vi "GEA_ICP_SM.vi"(0 "ComPort":refnum<visa-resource-name>="COM1", 1 "Destination Address":u8=96 format="%.0x", 2 "Source Address":u8=128 format="%.0x", 5 "Command":u8(ring)=15 items=["CMD_WRITE_SETPOINTS", "RQST_NON_CRIT_VERSION", "RQST_CRIT_VERSION", "RQST_EEPROM_VERSION", "RQST_T2_RESISTANCE", "RQST_T3A_RESISTANCE", "RQST_T3B_RESISTANCE", "RQST_T4_RESISTANCE", "RQST_T5_RESISTANCE", "RQST_IDLB_RESISTANCE", "RQST_MODE_SELECT_RESISTANCE", "RQST_STATUS INFO", "RQST_SS_FAULT_COUNTS", "RQST_OTHER_FAULT_COUNTS", "CMD_CLEAR_FAULT_COUNTS", "RQST_HYPERTERM_OUTPUT_DATA", "RQST_READ_PERSONALITY", "RQST_DSM_OVERRIDE_STATUS", "RQST_STATUS_QUERY", "RQST_HEM_KWH_DATA", "RQST_SERVICE_ERROR_CODES", "RQST_OVERRIDE_STATUS", "CMD_CLEAR_OVERRIDE_STATUS", "CMD_CLEAR_ENERGY_USAGE_CTRS", "CMD_COMP_OFF", "CMD_UE_2_SECONDS", "CMD_LE_2_SECONDS", "CMD_COMP_ON", "CMD_HP_RUN_6MIN", "RQST_TEMP_RANGE", "RQST_VACATION_RANGE", "RQST_STD_ELEC_RANGE", "RQST_WATER_CAPACITY", "CMD_CANCEL_EEV_POSITION", "RQST_SUPPORTED_MODES", "CMD_CONTROL_FAN1", "CMD_EEV_POSITION", "CMD_SET_EEV_START_POSITION", "CMD_SET_EEV_STOP_POSITION", "CMD_UPDATE_DSM_LEVEL", "CMD_SET_PID_I_DENOMINATOR", "CMD_SET_PID_I_NUMERATOR", "RQST_DATA_FROM_MEMORY", "CMD_OVERRIDE_STATUS_CHANGED", "CMD_SET_PID_P_DENOMINATOR", "CMD_SET_PID_P_NUMERATOR", "CMD_SET_PID_RUN_SH_TARGET", "CMD_SET_PID_START_DWELL_TIME", "CMD_SET_PID_TRANSITION_TIME", "CMD_SET_PID_TRANS_SH_TARGET", "CMD_SET_PID_UPDATE_RATE", "RQST_DATA_FROM_DATA_FLASH", "CMD_DSM_OVERRIDES", "CMD_UPDATE_MODE", "CMD_UPDATE_SPECIAL_OPERATION", "CMD_SET_CURRENTS", "CMD_RESET_FILTER_TIMES", "CMD_TURN_ON_DLB", "RQST_PID_PARAMETERS", "CMD_CHECK_CRC", "CMD_ENTER_FACT_MODE", "CMD_RESET", "CMD_RESTORE_EEPROM_DEFAULTS"], 7 "Command Data":u8[](array[numeric]) format="%02x", 9 "InitSerial?":bool=TRUE, 11 "Error In":errorcluster) -> (4 "WriteACK":bool, 6 "Read_ACK":bool, 8 "DataReturned":u8[](array[numeric]) format="%.0x", 14 "CRC Match":bool, 15 "Error Out":errorcluster)   [LabVIEW 2009]
uses:
  <vilib>/Instr/_visa.llb/VISA Configure Serial Port (Instr).vi
  HEWH Error Enumeration.ctl
panel:
  in  "milliseconds to wait":u32=20
  out "Numeric":i32
  out "Serial Settings:Number of Bytes at Serial Port 4":u32
  out "byte count":u32=40
  out "Serial Settings:Number of Bytes at Serial Port 3":u32
  out "Serial Settings:Number of Bytes at Serial Port 2":u32
  out "tStart":u32
  out "Tdiff":i32[](array[numeric])
  out "Serial Settings:Number of Bytes at Serial Port":u32
  out "Time Array":i32[](array[numeric])
  out "ACK(E1?)":u8[](array[numeric]) format="%.0x"
  out "Local?":bool
  out "State Array":string[](array[string])
  out "CRCRead":u8[](array[numeric]) format="%.0x"
  out "Command":u8[](array[numeric])=[226, 96, 8, 128, 86, 123, 137, 227] format="%.0x"
  in  "Send HEWH Cmd":bool
  in  "Write Rand":bool
  in  "Random Data":u8[](array[numeric]) format="%.0x"
  out "WriteOK":bool
  out "ReadArray":u8[](array[numeric]) format="%.0x"
  in  "OK":bool
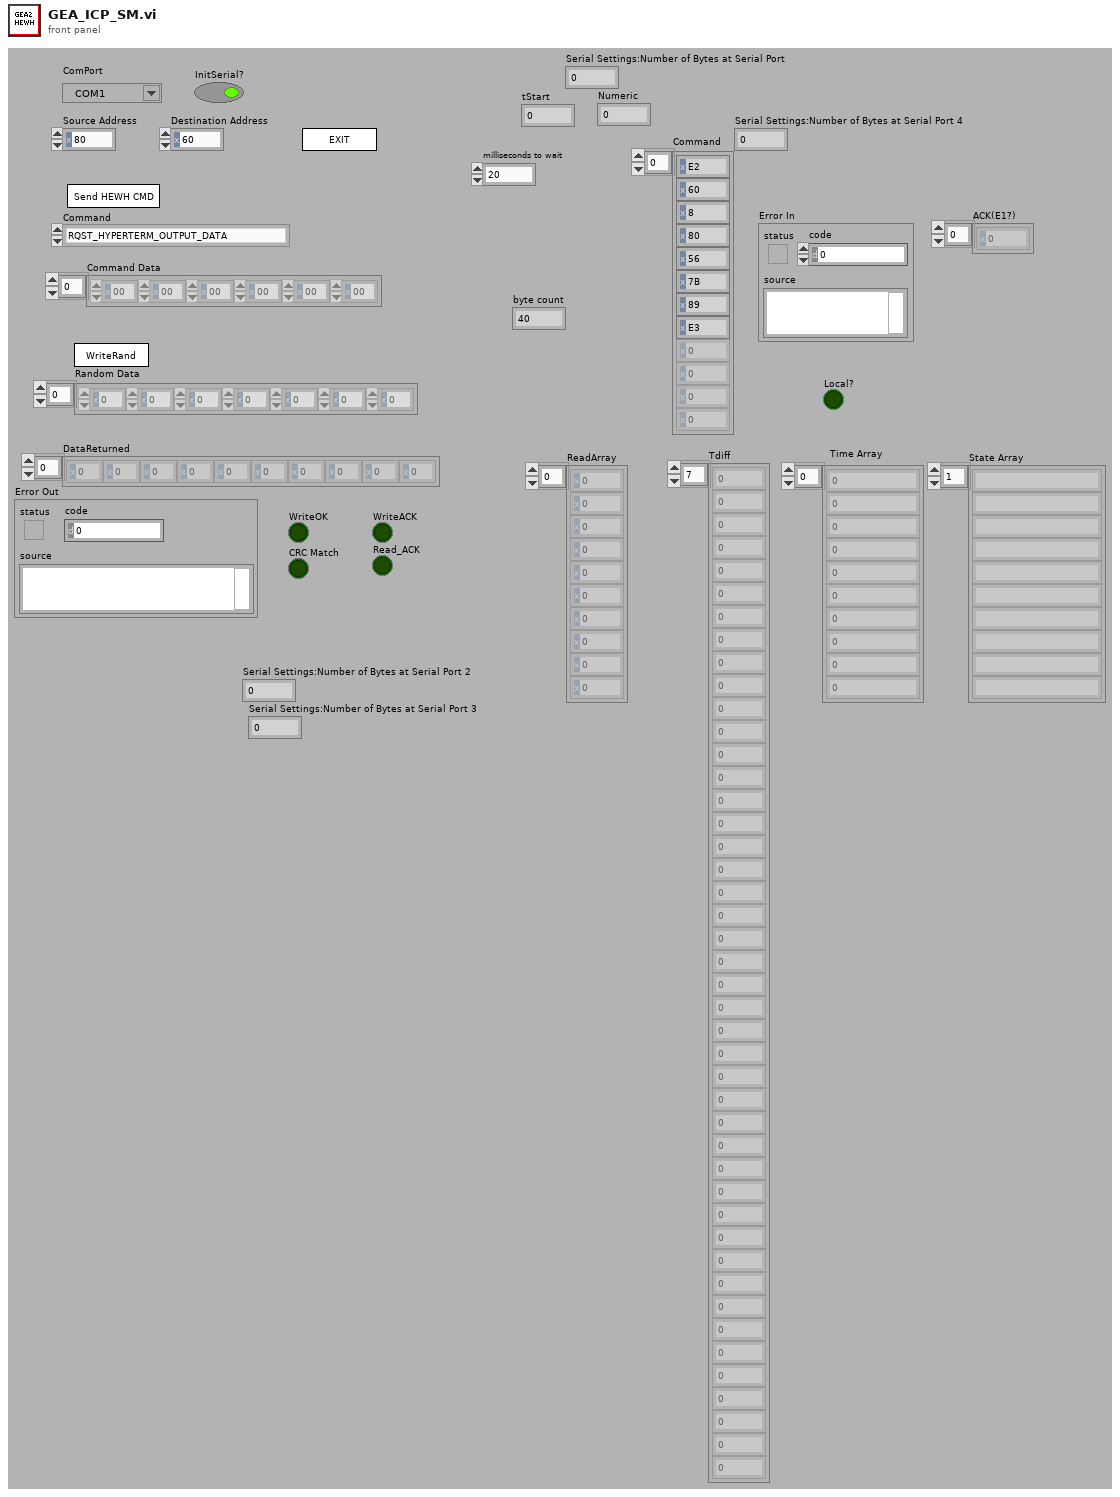
[diagram p1: front panel]
types:
  T1 = enum32{"invalid app kind", "Development System", "Run Time System", "Student Edition", "Embedded LabVIEW", "Evaluation", "Custom"}
  T2 = cluster{"Current VI Reference":refnum<vi>, "Close Panel on Exit?":bool}
  T3 = enum32{"Invalid", "Standard", "Closed", "Hidden", "Minimized", "Maximized"}
  T4 = typedef "HEWH Error Enumeration.ctl" = enum16{"No Error", "GEA2 Send ACK Mismatch", "GEA2 STX", "GEA2 ETX", "GEA2 CRC Mismatch", "GEA2 ReadACK", "RTD In Range Error", "Fail Mean Tank Temp", "No Flow Config Data Found", "Failed Flow During Purge", "Temp During Purge", "Confirm IF Stop Fail", "Init Draw: TC_1 Out of Range", "Flow = 0 During Draw after 20s"}
  T5 = cluster{"Core":cluster{"Current VI Reference":refnum<vi>, "Close Panel on Exit?":bool}, "ComPort":refnum<visa-resource-name>, "ReadArray":u8[], "CRCArray":u8[], "Bytes Remaining":u8, "CRCRead":u8[], "CRC":bool, "HEWH Command":u8, "Error Out Flag":bool, "Read Pos.":i32}
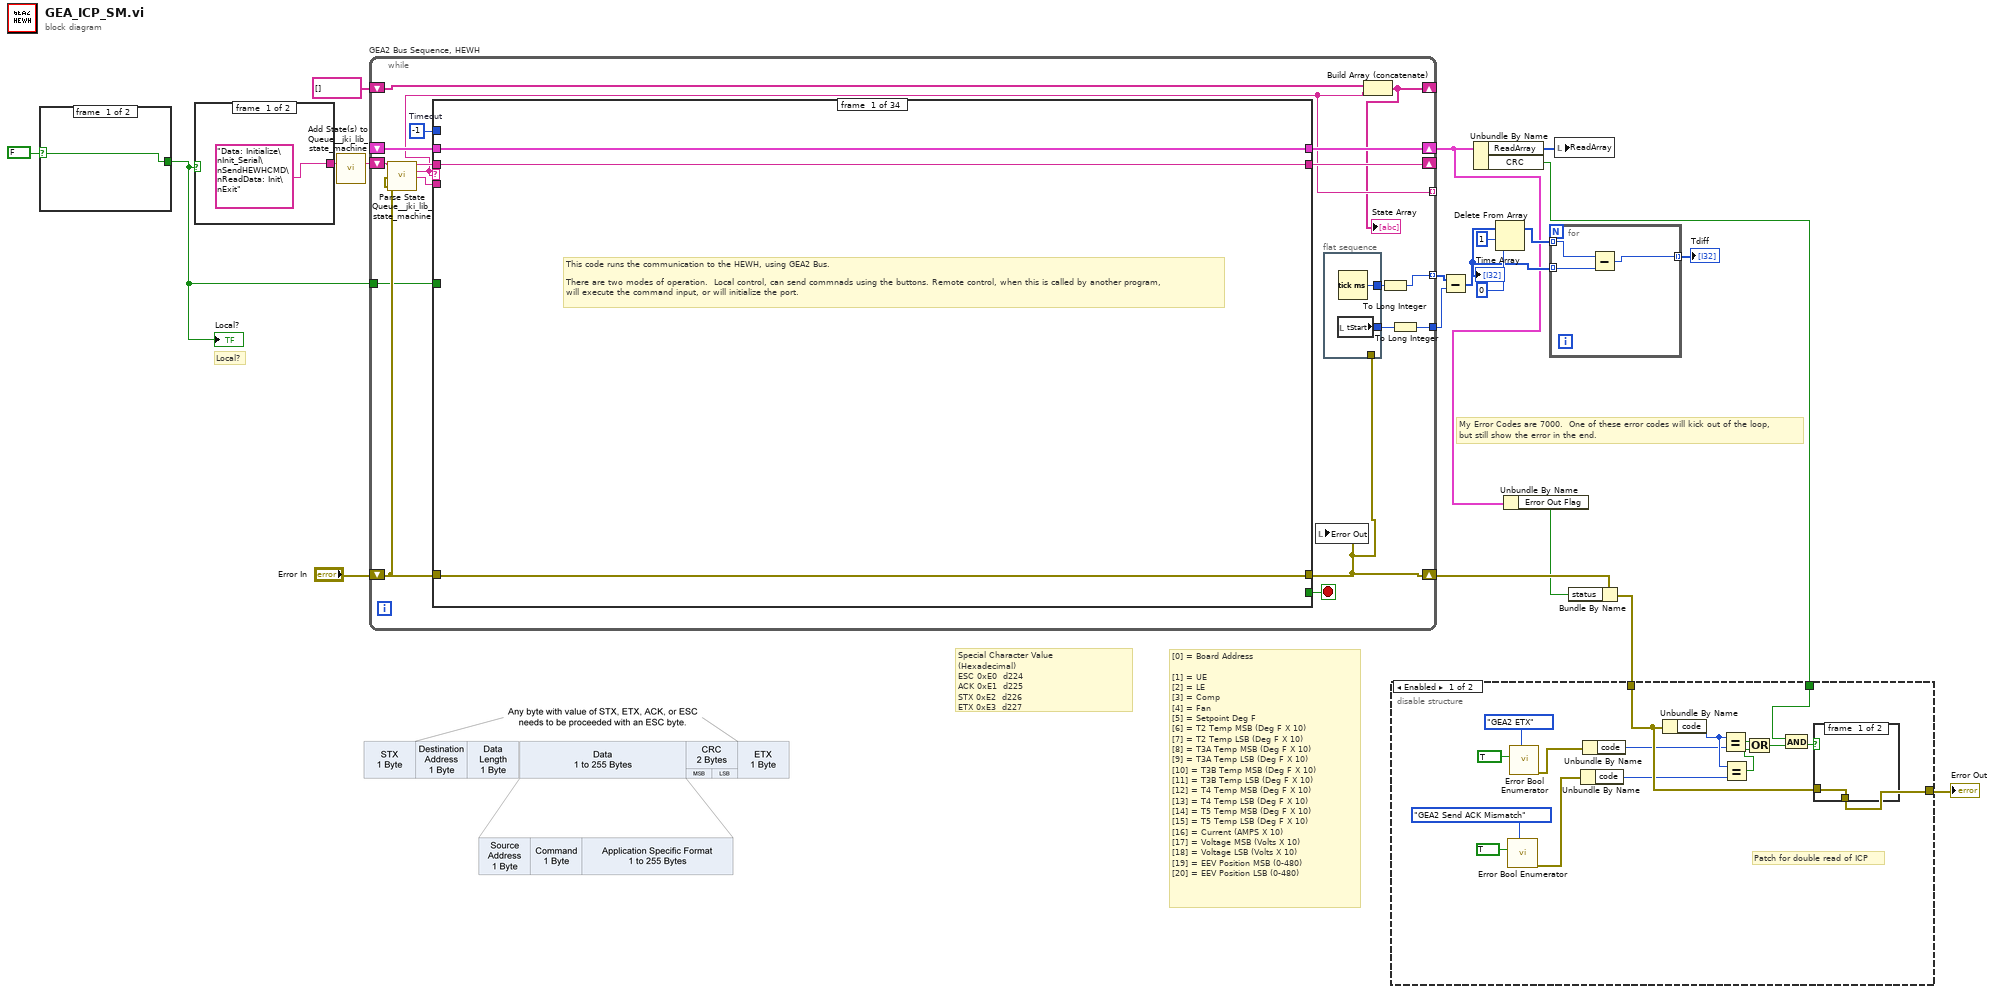
[diagram p0: block diagram]
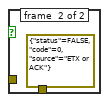
[diagram p2: hidden frame]
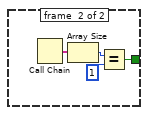
[diagram p4: hidden frame]
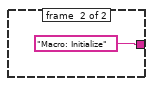
[diagram p5: hidden frame]
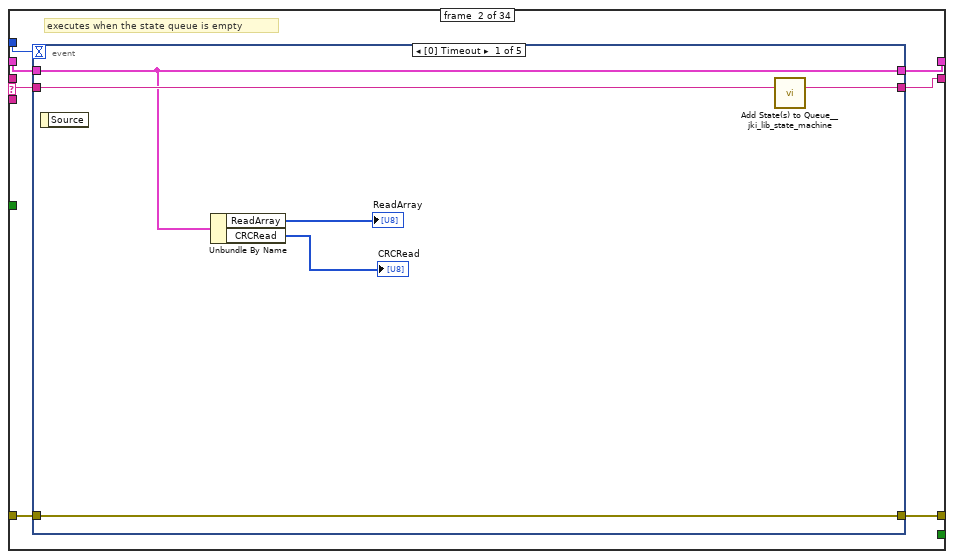
[diagram p6: hidden frame]
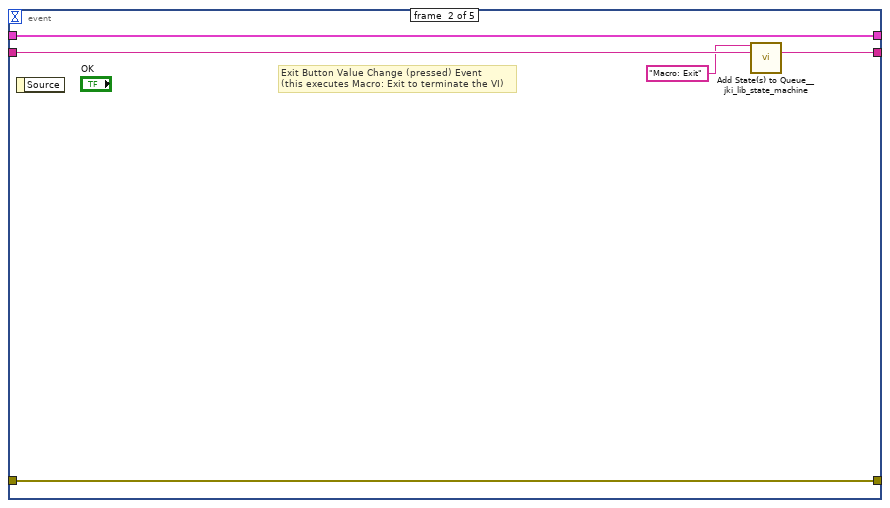
[diagram p7: hidden frame]
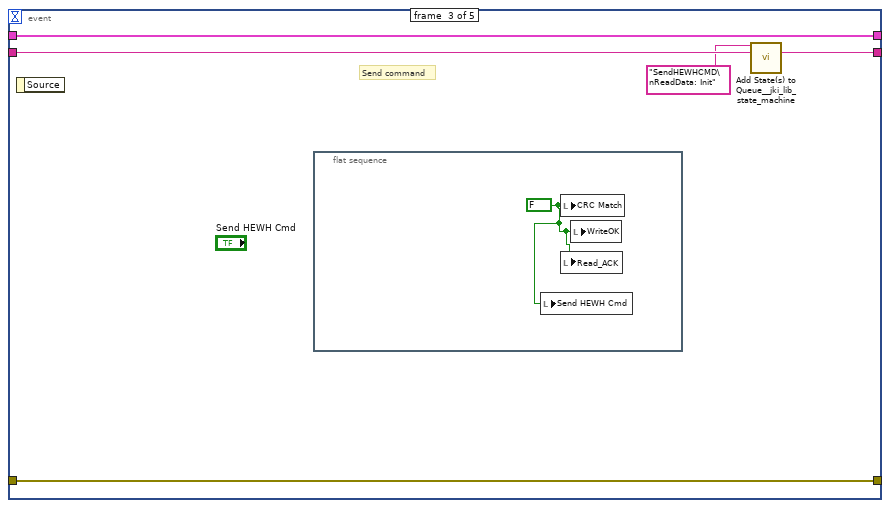
[diagram p8: hidden frame]
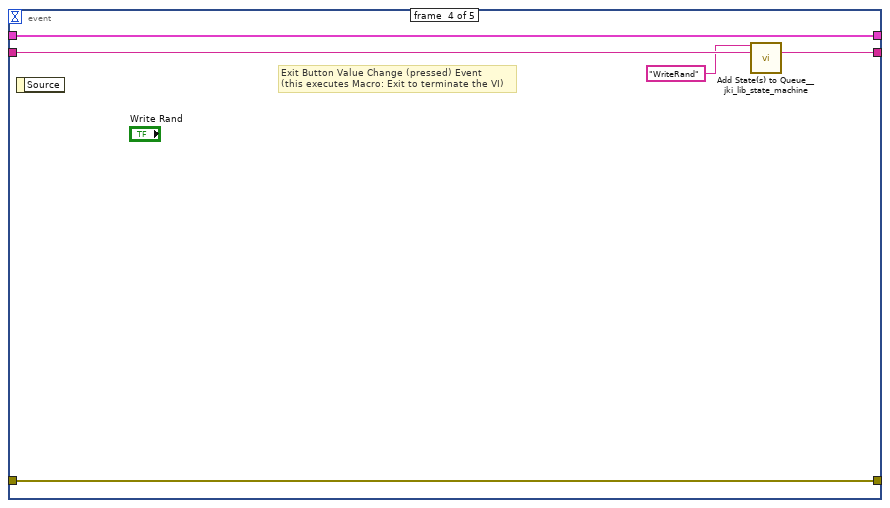
[diagram p9: hidden frame]
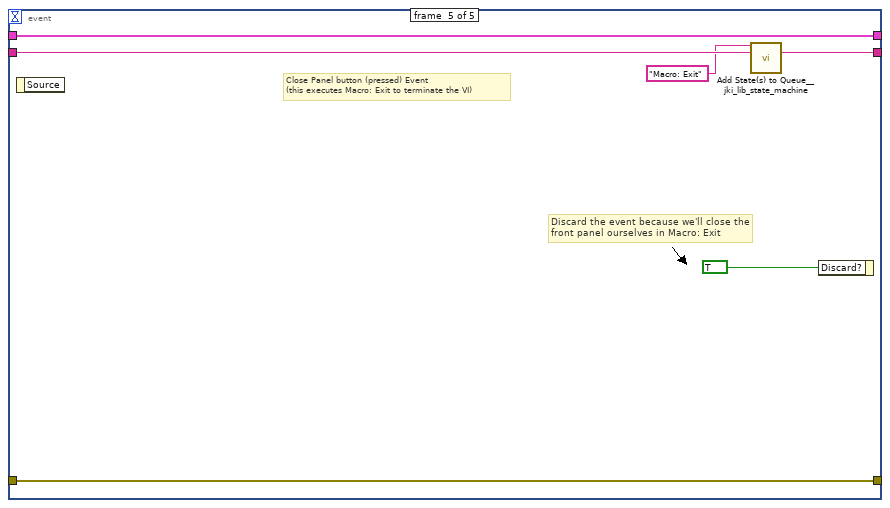
[diagram p10: hidden frame]
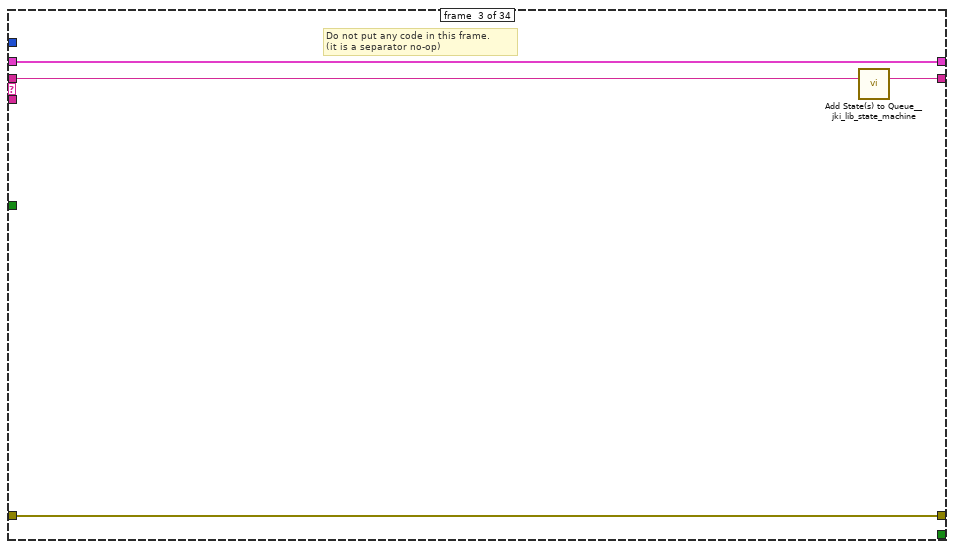
[diagram p11: hidden frame]
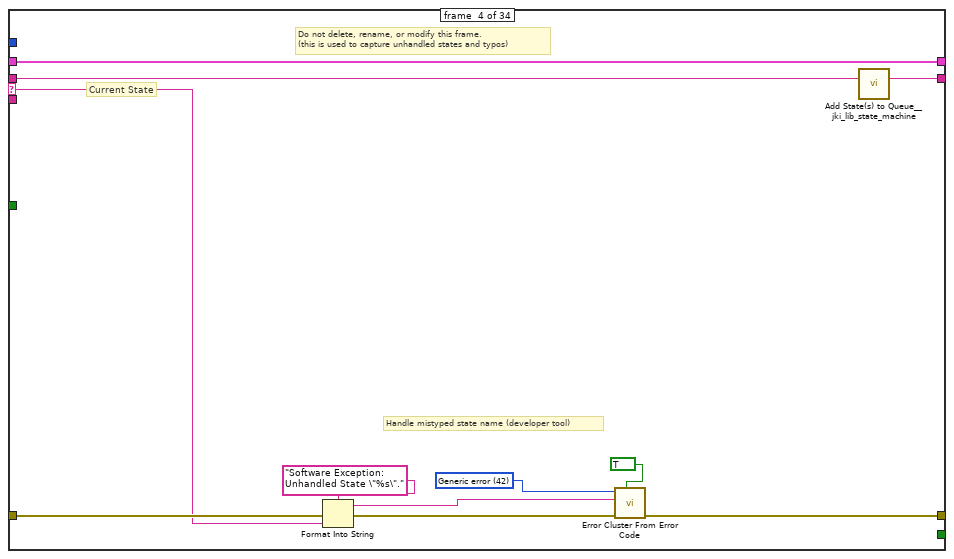
[diagram p12: hidden frame]
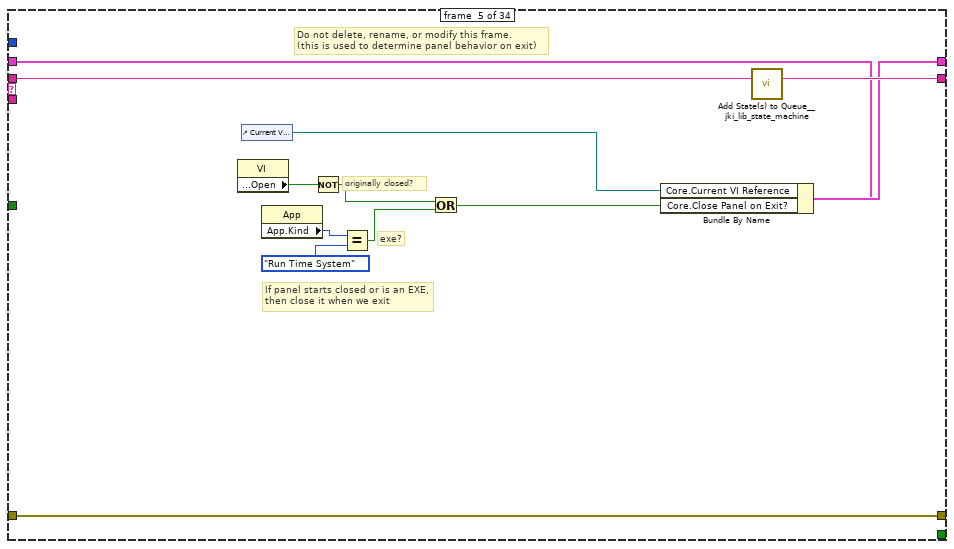
[diagram p13: hidden frame]
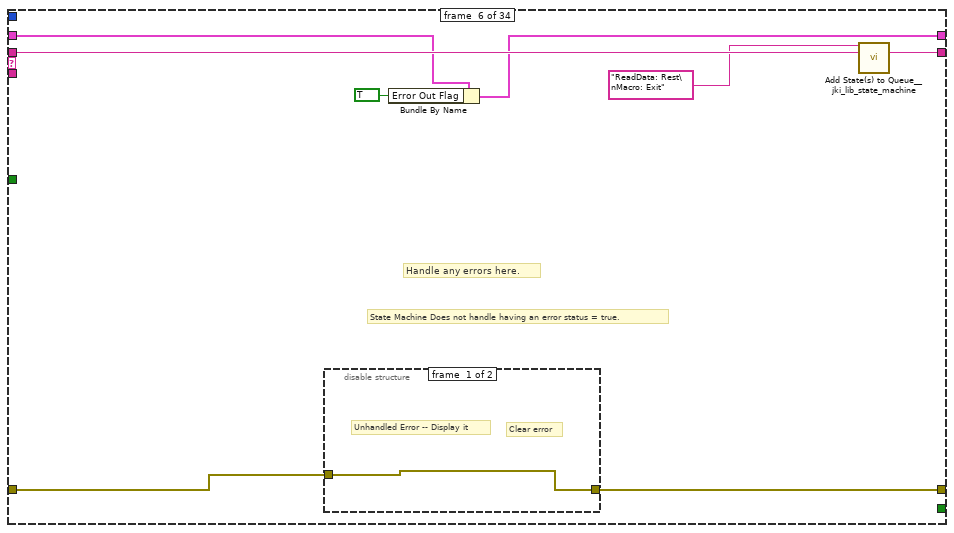
[diagram p14: hidden frame]
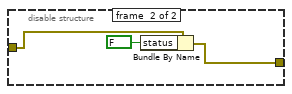
[diagram p15: hidden frame]
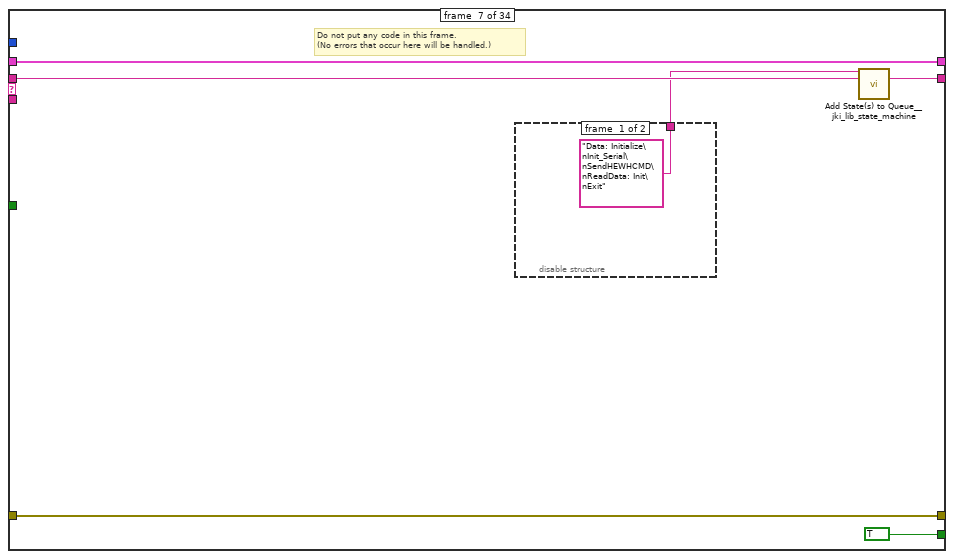
[diagram p16: hidden frame]
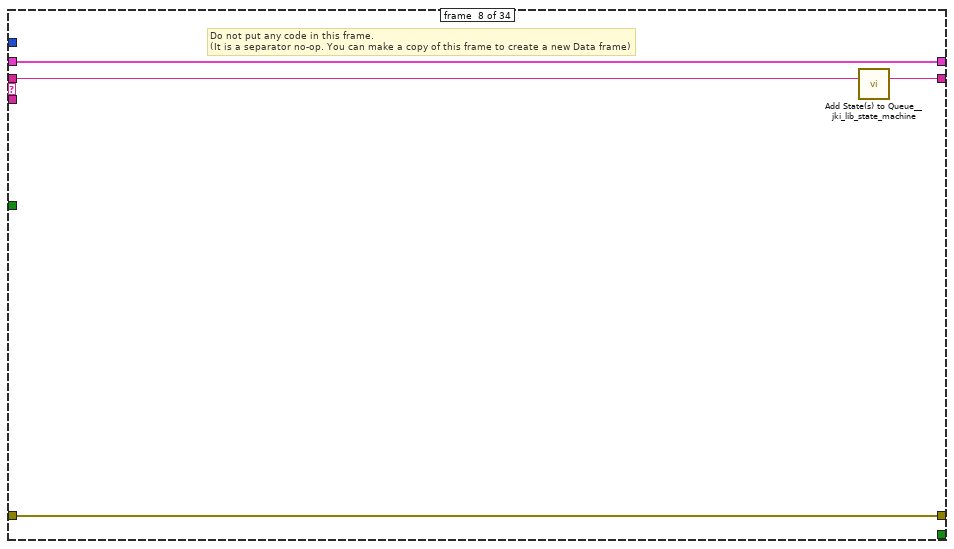
[diagram p18: hidden frame]
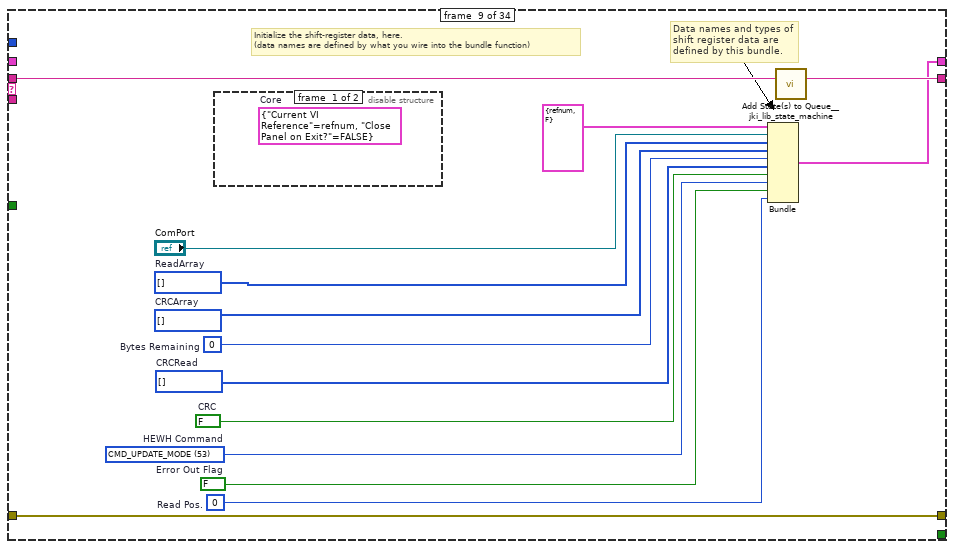
[diagram p19: hidden frame]
diagram:
  # "My Error Codes are 7000.  One of these error codes will kick out of the loop,\nbut still show the error in the end."
  # "Local?"
  # "Special Character\tValue (Hexadecimal)\nESC\t0xE0  d224\nACK\t0xE1  d225\nSTX\t0xE2  d226\nETX\t0xE3  d227"
  # "[0] = Board Address\n\n[1] = UE\n[2] = LE\n[3] = Comp\n[4] = Fan\n[5] = Setpoint Deg F\n[6] = T2 Temp MSB (Deg F X 10)\n[7] = T2 Temp LSB (Deg F X 10)\n[8] = T3A Temp MSB (Deg F X 10)\n[9] = T3A Temp LSB (Deg F X 10)\n[10] = T3B Temp MSB (Deg F X 10)\n[11] = T3B Temp LSB (Deg F X 10)\n[12] = T4 Temp MSB (Deg F X 10)\n[13] = T4 Temp LSB (Deg F X 10)\n[14] = T5 Temp MSB (Deg F X 10)\n[15] = T5 Temp LSB (Deg F X 10)\n[16] = Current (AMPS X 10)\n[17] = Voltage MSB (Volts X 10)\n[18] = Voltage LSB (Volts X 10)\n[19] = EEV Position MSB (0-480)\n[20] = EEV Position LSB (0-480)"
  n1 = case shown="True" FALSE {
    selector: FALSE -> [w21 _]
    tunnel: [w21 w22] -> w17
    frame #0 {
    }
    frame #1 {
      n2 = Call Chain() -> (call chain=w25:string[])
      n3 = Array Size(array=w25) -> (size(s)=w24:i32)
      n4 = Equal?(x=w24, y=1) -> (x = y?=w22:bool)
    }
  }
  "Local?" <- w17
  n5 = case shown="False" w17 {
    tunnel: ["Data: Initialize\nInit_Serial\nSendHEWHCMD\nReadData: Init\nExit" "Macro: Initialize"] -> w19
    frame #0 {
    }
    frame #1 {
    }
  }
  n6 = call <vilib>:"Add State(s) to Queue__jki_lib_state_machine.vi"("State(s) in (\"\")"=w19) -> ("States Out"=w20:string)  [unwired: 14 in]
  n7 = while "GEA2 Bus Sequence, HEWH" {
    shift-right: [w41] -> w2
    shift-left: _ -> [w40]
    shift-right: [w35] -> w16
    shift-left: "Error In" -> [w38]
    shift-right: [w36] -> _
    shift-left: w20 -> [w43]
    tunnel: w17 -> [w37]
    tunnel: [w29] -> _ mode=indexing
    tunnel: [w32] -> w10 mode=indexing
    tunnel: [w31] -> w9
    shift-right: [w28] -> _
    shift-left: string[] [] -> [w30]
    stop <- w42 stop-if-true
    w39 = -1  # Timeout
    n8 = call <vilib>:"Parse State Queue__jki_lib_state_machine.vi"("State Queue"=w43, "Error In (no error)"=w38) -> ("Remaining States"=w45:string, "Current State"=w29:string, "Arguments"=w44:string)  [unwired: 11 in]
    n9 = case shown="\"ReadData: Init\"" w29 {
      selector: w29 -> [_ _ _ w90 _ _ _ _ _ _ _ _ _ _ _ _ _ _ _ _ _ _ _ _ _ _ _ _ _ _ _ _ _ _]
      tunnel: w45 -> [w49 w57 w89 w94 w112 w120 w130 w135 w149 w155 w164 w169 w175 w186 w212 w217 w222 w233 w242 w360 w389 w404 w413 w449 w484 w531 w575 w613 w647 w671 w700 w725 w746 w774]
      tunnel: w44 -> [_ _ _ _ _ _ _ _ _ _ _ _ w170 w180 _ _ _ _ _ _ _ _ _ _ _ _ _ _ _ _ _ _ _ _]
      tunnel: w40 -> [w50 w55 w86 w92 w103 w115 w128 w132 _ w152 w161 w167 w173 w182 w209 w214 w219 w230 w239 w334 w387 w401 w407 w446 w482 w528 w572 w610 w645 w662 w681 w720 w743 w754]
      tunnel: [w48 w54 w87 w96 w109 w118 w127 w133 w146 w150 w162 w166 w171 w183 w210 w215 w220 w231 w240 w331 w383 w402 w411 w436 w474 w521 w567 w594 w631 w666 w692 w715 w733 w757] -> w35
      tunnel: w38 -> [w48 w53 w87 w95 w109 w117 w127 w133 w146 w153 w162 w166 w172 w184 w210 w215 w220 w231 w237 w336 w384 w402 w411 w439 w476 w523 w568 w606 w641 w668 w695 w718 w735 w772]
      tunnel: [w49 w56 w88 w93 w111 w119 w129 w134 w148 w154 w163 w168 w174 w185 w211 w216 w221 w232 w241 w359 w388 w403 w412 w448 w483 w530 w574 w612 w646 w670 w699 w724 w745 w773] -> w36
      tunnel: [_ _ _ _ _ _ TRUE _ _ _ _ _ _ _ _ _ _ _ _ _ _ _ _ _ _ _ _ _ _ _ _ _ _ _] -> w42
      tunnel: [w50 w52 w86 w92 w110 w114 w128 w132 w147 w152 w161 w167 w173 w182 w209 w214 w219 w230 w238 w333 w387 w401 w410 w445 w481 w527 w571 w609 w644 w661 w696 w719 w742 w753] -> w41
      tunnel: w39 -> [_ w51 _ _ _ _ _ _ _ _ _ _ _ _ _ _ _ _ _ _ _ _ _ _ _ _ _ _ _ _ _ _ _ _]
      tunnel: w37 -> [_ _ _ _ _ _ _ _ _ w151 _ _ _ _ _ _ _ _ w236 _ _ _ _ _ _ _ _ _ _ _ _ _ _ _]
      frame #0 {
        # "This code runs the communication to the HEWH, using GEA2 Bus.\n\nThere are two modes of operation.  Local control, can send commnads using the buttons. Remote control, when this is called by another program,\nwill execute the command input, or will initialize the port."
      }
      frame #1 {
        # "executes when the state queue is empty"
        n10 = event shown="[0] Timeout" {
          selector: _ -> [_ _ _ _ _]
          dyn-events: _ -> [_ _ _ _ _]
          timeout: w51 -> [_ _ _ _ _]
          tunnel: w57 -> [w63 w68 w73 w79 w85]
          tunnel: [w62 w67 w72 w78 w84] -> w56
          tunnel: w55 -> [w60 w65 w70 w76 w82]
          tunnel: [w61 w66 w71 w77 w83] -> w54
          tunnel: w53 -> [w61 w66 w71 w77 w83]
          tunnel: [w60 w65 w70 w76 w82] -> w52
          event #0 {
            n11 = event-data() -> ()  [unwired: 1 in, 1 out]
            n12 = Unbundle By Name(w60) -> ("ReadArray"=→"ReadArray":u8[], "CRCRead"=→"CRCRead":u8[])
            n13 = call <vilib>:"Add State(s) to Queue__jki_lib_state_machine.vi"("State(s) in (\"\")"=w63) -> ("States Out"=w62:string)  [unwired: 14 in]
          }
          event #1 {
            # "Exit Button Value Change (pressed) Event\n(this executes Macro: Exit to terminate the VI)"
            n14 = event-data() -> ()  [unwired: 1 in, 1 out]
            n15 = call <vilib>:"Add State(s) to Queue__jki_lib_state_machine.vi"("State(s) in Front (\"\")"="Macro: Exit", "State(s) in (\"\")"=w68) -> ("States Out"=w67:string)  [unwired: 13 in]
          }
          event #2 {
            # "Send command"
            n16 = event-data() -> ()  [unwired: 1 in, 1 out]
            n17 = flat-sequence {
              frame #0 {
                w74 = FALSE ("CRC Match")
                n18 = local write "Send HEWH Cmd"(w74) -> ()
                n19 = local write "CRC Match"(w74) -> ()
                n20 = local write "Read_ACK"(w74) -> ()
                n21 = local write "WriteOK"(w74) -> ()
              }
            }
            n22 = call <vilib>:"Add State(s) to Queue__jki_lib_state_machine.vi"("State(s) in Front (\"\")"="SendHEWHCMD\nReadData: Init", "State(s) in (\"\")"=w73) -> ("States Out"=w72:string)  [unwired: 13 in]
          }
          event #3 {
            # "Exit Button Value Change (pressed) Event\n(this executes Macro: Exit to terminate the VI)"
            n23 = event-data() -> ()  [unwired: 1 in, 1 out]
            n24 = call <vilib>:"Add State(s) to Queue__jki_lib_state_machine.vi"("State(s) in Front (\"\")"="WriteRand", "State(s) in (\"\")"=w79) -> ("States Out"=w78:string)  [unwired: 13 in]
          }
          event #4 {
            # "Discard the event because we'll close the front panel ourselves in Macro: Exit"
            # "Close Panel button (pressed) Event\n(this executes Macro: Exit to terminate the VI)"
            n25 = event-data() -> ()  [unwired: 1 in, 1 out]
            n26 = call <vilib>:"Add State(s) to Queue__jki_lib_state_machine.vi"("State(s) in Front (\"\")"="Macro: Exit", "State(s) in (\"\")"=w85) -> ("States Out"=w84:string)  [unwired: 13 in]
            n27 = event-data("Discard?"=TRUE) -> ()  [unwired: 1 in, 1 out]
          }
        }
      }
      frame #2 {
        # "Do not put any code in this frame.\n(it is a separator no-op)"
        n28 = call <vilib>:"Add State(s) to Queue__jki_lib_state_machine.vi"("State(s) in (\"\")"=w89) -> ("States Out"=w88:string)  [unwired: 14 in]
      }
      frame #3 {
        w99 = 42 items=["No error", "Argument error", "Memory is full", "Out of zone", "End of file", "File already open", "Generic file I/O error", "File not found", "File permission error", "Disk is full", "Duplicate path", "Too many files open", "System feature not enabled", "Resource file not found", "Cannot add resource", "Resource not found", "Image not found", "Image memory error", "Pen does not exist", "Config type invalid", "Config token not found", "Config parse error", "Config memory error", "Bad external code format", "Bad external code offset", "External code not present", "Null window", "Destroy window error", "Null menu", "Print aborted", "Bad print record", "Print driver error", "Windows error during printing", "Memory error during printing", "Print dialog error", "Generic print error", "Invalid device refnum", "Device not found", "Device parameter error", "Device unit error", "Cannot open device", "Device call aborted", "Generic error", "Cancelled by user", "Object ID too low", "Object ID too high", "Object not in heap", "Unknown heap", "Unknown object (invalid DefProc)", "Unknown object (DefProc not in table)", "Message out of range", "Invalid (null) method", "Unknown message", "Manager call not supported", "Bad address", "Network operation in progress", "Network operation timed out", "Connection is busy", "Network attribute not supported", "Network error", "Address in use", "System out of memory", "Connection aborted", "Connection refused", "Not connected", "Already connected", "Connection closed", "Initialization error (interapplication manager)", "Bad occurrence", "Wait on unbound occurrence handler", "Occurrence queue overflow", "Datalog type conflict", "Unused", "Unrecognized type (interapplication manager)", "Memory corrupt", "Failed to make temporary DLL", "Old CIN version", "Drag socket not found", "Failed to load drop-object", "Failed to register OLE object", "Failed to release OLE object", "Format specifier type mismatch", "Unknown format specifier", "Too few format specifiers", "Too many format specifiers", "Scan failed", "Newer CIN version", "Error converting to variant", "Runtime menu error", "Password tampered", "Variant attribute not found", "Incompatible variant data type", "Event data is not available", "Event Store is not present", "Occurrence is not found", "Event Queue is not created", "Event info is not available", "Refnum passed is NULL", "Error retrieving Class GUID", "Error retrieving CoClass GUID", "Error retrieving TypeLib GUID.", "Bad built application magic bytes.", "Specific driver is different from the specific driver associated with the Logical Name.", "There is no session opened to the class driver.", "Max Error", "MAX - Error with config objects", "MAX - Error loading configuration", "MAX - Group not supported"]
        # "Current State"
        # "Do not delete, rename, or modify this frame.\n(this is used to capture unhandled states and typos)"
        # "Handle mistyped state name (developer tool)"
        n29 = Format Into String(format string="Software Exception: Unhandled State \"%s\"." ("message"), error in=w95, w90) -> (resulting string=w98:string, error out=w97:errorcluster)  [unwired: 1 in]
        n30 = call <vilib>:"Error Cluster From Error Code.vi"("show call chain? (False)"=TRUE, "error in (no error)"=w97, "error message (\"\")"=w98, "error code (0)"=w99) -> ("error out"=w96:errorcluster)  [unwired: 5 in]
        n31 = call <vilib>:"Add State(s) to Queue__jki_lib_state_machine.vi"("State(s) in (\"\")"=w94) -> ("States Out"=w93:string)  [unwired: 14 in]
      }
      frame #4 {
        # "Do not delete, rename, or modify this frame.\n(this is used to determine panel behavior on exit)"
        # "originally closed?"
        # "exe?"
        # "If panel starts closed or is an EXE, then close it when we exit"
        n32 = property class="VI"() -> ("Front Panel.Open"=w108:bool)  [unwired: 2 in, 2 out]
        n33 = control-ref of="Current VI Reference"() -> (w101:refnum<vi>)
        n34 = property class="App"() -> ("App.Kind"=w107:T1)  [unwired: 2 in, 2 out]
        n35 = Not(x=w108) -> (.not. x?=w105:bool)
        n36 = Equal?(x=w107, y=T1."Run Time System" ("Application:Kind")) -> (x = y?=w104:bool)
        n37 = Or(x=w105, y=w104) -> (x .or. y?=w102:bool)
        n38 = Bundle By Name(cluster=w103, "Core.Current VI Reference"=w101, "Core.Close Panel on Exit?"=w102) -> (w110:T5)
        n39 = call <vilib>:"Add State(s) to Queue__jki_lib_state_machine.vi"("State(s) in (\"\")"=w112) -> ("States Out"=w111:string)  [unwired: 14 in]
      }
      frame #5 {
        # "State Machine Does not handle having an error status = true."
        # "Handle any errors here."
        n40 = disable-structure shown="Enabled" {
          disable-tunnel: [w121 w123] -> w118
          disable-tunnel: w117 -> [w121 w124]
          frame #0 {
            # "Unhandled Error -- Display it"
            # "Clear error"
          }
          frame #1 {
            n41 = Bundle By Name(cluster=w124, "status"=FALSE) -> (w123:errorcluster)
          }
        }
        n42 = Bundle By Name(cluster=w115, "Error Out Flag"=TRUE) -> (w114:T5)
        n43 = call <vilib>:"Add State(s) to Queue__jki_lib_state_machine.vi"("State(s) in Front (\"\")"="ReadData: Rest\nMacro: Exit", "State(s) in (\"\")"=w120) -> ("States Out"=w119:string)  [unwired: 13 in]
      }
      frame #6 {
        # "Do not put any code in this frame.\n(No errors that occur here will be handled.)"
        n44 = disable-structure shown="Enabled" {
          disable-tunnel: ["Data: Initialize\nInit_Serial\nSendHEWHCMD\nReadData: Init\nExit" _] -> w125
          frame #0 {
          }
          frame #1 {
          }
        }
        n45 = call <vilib>:"Add State(s) to Queue__jki_lib_state_machine.vi"("State(s) in Front (\"\")"=w125, "State(s) in (\"\")"=w130) -> ("States Out"=w129:string)  [unwired: 13 in]
      }
      frame #7 {
        # "Do not put any code in this frame.\n(It is a separator no-op. You can make a copy of this frame to create a new Data frame)"
        n46 = call <vilib>:"Add State(s) to Queue__jki_lib_state_machine.vi"("State(s) in (\"\")"=w135) -> ("States Out"=w134:string)  [unwired: 14 in]
      }
      frame #8 {
        w136 = 0  # Read Pos.
        w137 = FALSE  # Error Out Flag
        w138 = u8 53 items=["CMD_WRITE_SETPOINTS", "RQST_NON_CRIT_VERSION", "RQST_CRIT_VERSION", "RQST_EEPROM_VERSION", "RQST_T2_RESISTANCE", "RQST_T3A_RESISTANCE", "RQST_T3B_RESISTANCE", "RQST_T4_RESISTANCE", "RQST_T5_RESISTANCE", "RQST_IDLB_RESISTANCE", "RQST_MODE_SELECT_RESISTANCE", "RQST_STATUS INFO", "RQST_SS_FAULT_COUNTS", "RQST_OTHER_FAULT_COUNTS", "CMD_CLEAR_FAULT_COUNTS", "RQST_HYPERTERM_OUTPUT_DATA", "RQST_READ_PERSONALITY", "RQST_DSM_OVERRIDE_STATUS", "RQST_STATUS_QUERY", "RQST_HEM_KWH_DATA", "RQST_SERVICE_ERROR_CODES", "RQST_OVERRIDE_STATUS", "CMD_CLEAR_OVERRIDE_STATUS", "CMD_CLEAR_ENERGY_USAGE_CTRS", "CMD_COMP_OFF", "CMD_UE_2_SECONDS", "CMD_LE_2_SECONDS", "CMD_COMP_ON", "CMD_HP_RUN_6MIN", "RQST_TEMP_RANGE", "RQST_VACATION_RANGE", "RQST_STD_ELEC_RANGE", "RQST_WATER_CAPACITY", "CMD_CANCEL_EEV_POSITION", "RQST_SUPPORTED_MODES", "CMD_CONTROL_FAN1", "CMD_EEV_POSITION", "CMD_SET_EEV_START_POSITION", "CMD_SET_EEV_STOP_POSITION", "CMD_UPDATE_DSM_LEVEL", "CMD_SET_PID_I_DENOMINATOR", "CMD_SET_PID_I_NUMERATOR", "RQST_DATA_FROM_MEMORY", "CMD_OVERRIDE_STATUS_CHANGED", "CMD_SET_PID_P_DENOMINATOR", "CMD_SET_PID_P_NUMERATOR", "CMD_SET_PID_RUN_SH_TARGET", "CMD_SET_PID_START_DWELL_TIME", "CMD_SET_PID_TRANSITION_TIME", "CMD_SET_PID_TRANS_SH_TARGET", "CMD_SET_PID_UPDATE_RATE", "RQST_DATA_FROM_DATA_FLASH", "CMD_DSM_OVERRIDES", "CMD_UPDATE_MODE", "CMD_UPDATE_SPECIAL_OPERATION", "CMD_SET_CURRENTS", "CMD_RESET_FILTER_TIMES", "CMD_TURN_ON_DLB", "RQST_PID_PARAMETERS", "CMD_CHECK_CRC", "CMD_ENTER_FACT_MODE", "CMD_RESET", "CMD_RESTORE_EEPROM_DEFAULTS"]  # HEWH Command
        w140 = FALSE  # CRC
        w141 = u8[] []  # CRCRead
        w142 = u8 0  # Bytes Remaining
        w143 = u8[] []  # CRCArray
        w144 = u8[] []  # ReadArray
        # "Data names and types of shift register data are defined by this bundle."
        # "Initialize the shift-register data, here.\n(data names are defined by what you wire into the bundle function)"
        n47 = disable-structure shown="Enabled" {
          frame #0 {
            (unwired) T2 {"Current VI Reference"=refnum, "Close Panel on Exit?"=FALSE}  # Core
          }
          frame #1 {
          }
        }
        n48 = Bundle("Core"=T2 {"Current VI Reference"=refnum, "Close Panel on Exit?"=FALSE}, "ComPort"="ComPort", "ReadArray"=w144, "CRCArray"=w143, "Bytes Remaining"=w142, "CRCRead"=w141, "CRC"=w140, "HEWH Command"=w138, "Error Out Flag"=w137, "Read Pos."=w136) -> (w147:T5)  [unwired: 1 in]
        n49 = call <vilib>:"Add State(s) to Queue__jki_lib_state_machine.vi"("State(s) in (\"\")"=w149) -> ("States Out"=w148:string)  [unwired: 14 in]
      }
      frame #9 {
        # "Cleanup any data and references, here.\n(this is called automatically, by the Macro: Exit)"
        n50 = case shown="True" w151 {
          tunnel: w153 -> [w156 w159]
          tunnel: [w156 w158] -> w150
          tunnel: w152 -> [_ w157]
          frame #0 {
          }
          frame #1 {
            n51 = Unbundle By Name(w157) -> ("Core.Current VI Reference"=w160:refnum<vi>)
            n52 = Close Reference(reference=w160, error in (no error)=w159) -> (error out=w158:errorcluster)
          }
        }
        n53 = call <vilib>:"Add State(s) to Queue__jki_lib_state_machine.vi"("State(s) in (\"\")"=w155) -> ("States Out"=w154:string)  [unwired: 14 in]
      }
      frame #10 {
        # "Do not put any code in this frame.\n(It is a separator no-op. You can make a copy of this frame to create a new UI frame)"
        n54 = call <vilib>:"Add State(s) to Queue__jki_lib_state_machine.vi"("State(s) in (\"\")"=w164) -> ("States Out"=w163:string)  [unwired: 14 in]
      }
      frame #11 {
        w165 = FALSE ("CRC Match")
        # "Initialize the User Interface, here.\n(this is called automatically, by the Macro: Init)"
        n55 = local write "CRC Match"(w165) -> ()
        n56 = local write "WriteOK"(w165) -> ()
        n57 = local write "WriteACK"(w165) -> ()
        n58 = local write "Send HEWH Cmd"(w165) -> ()
        n59 = call <vilib>:"Add State(s) to Queue__jki_lib_state_machine.vi"("State(s) in (\"\")"=w169) -> ("States Out"=w168:string)  [unwired: 14 in]
      }
      frame #12 {
        # "Argument"
        # "Set and Unset Cursor Busy.\n(Usage: \"UI: Cursor Set >> Busy|Idle\")"
        n60 = case shown="\"Idle\", Default" w170 {
          tunnel: w172 -> [w177 w179]
          tunnel: [w176 w178] -> w171
          frame #0 {
            n61 = call <vilib>:"Unset Busy.vi"("error in (no error)"=w177) -> ("error out"=w176:errorcluster)  [unwired: 10 in]
          }
          frame #1 {
            n62 = call <vilib>:"Set Busy.vi"("error in (no error)"=w179) -> ("error out"=w178:errorcluster)  [unwired: 9 in, 1 out]
          }
        }
        n63 = call <vilib>:"Add State(s) to Queue__jki_lib_state_machine.vi"("State(s) in (\"\")"=w175) -> ("States Out"=w174:string)  [unwired: 14 in]
      }
      frame #13 {
        # "Argument"
        # "Set Front Panel Open or Closed\n(Usage: \"UI: Front Panel State >> Open|Close\")"
        n64 = Unbundle By Name(w182) -> ("Core.Current VI Reference"=w181:refnum<vi>)
        n65 = case shown="\"Close\"" w180 {
          tunnel: w184 -> [w190 w203]
          tunnel: [w192 w204] -> w183
          tunnel: w181 -> [w191 w201]
          frame #0 {
            n66 = property class="VI"(reference=w191, error in=w190) -> (reference out=w188:refnum<vi>, error out=w189:errorcluster, "Front Panel.Open"=w187:bool)
            n67 = case shown="False" w187 {
              tunnel: [w195 w198] -> w192
              tunnel: w189 -> [w194 w198]
              tunnel: w188 -> [w193 _]
              frame #0 {
                n68 = invoke class="VI" method="FP.Open"(reference=w193, error in=w194, "Activate"=TRUE, "State"=T3."Standard") -> (error out=w195:errorcluster)  [unwired: 1 in, 4 out]
              }
              frame #1 {
              }
            }
          }
          frame #1 {
            n69 = property class="VI"(reference=w201, error in=w203) -> (reference out=w200:refnum<vi>, error out=w202:errorcluster, "Front Panel.Open"=w199:bool)
            n70 = case shown="True" w199 {
              tunnel: [w205 w208] -> w204
              tunnel: w202 -> [w205 w207]
              tunnel: w200 -> [_ w206]
              frame #0 {
              }
              frame #1 {
                n71 = invoke class="VI" method="FP.Close"(reference=w206, error in=w207) -> (error out=w208:errorcluster)  [unwired: 1 in, 2 out]
              }
            }
          }
        }
        n72 = call <vilib>:"Add State(s) to Queue__jki_lib_state_machine.vi"("State(s) in (\"\")"=w186) -> ("States Out"=w185:string)  [unwired: 14 in]
      }
      frame #14 {
        # "Do not put any code in this frame.\n(It is a separator no-op. You can make a copy of this frame to create a new Macro frame)"
        n73 = call <vilib>:"Add State(s) to Queue__jki_lib_state_machine.vi"("State(s) in (\"\")"=w212) -> ("States Out"=w211:string)  [unwired: 14 in]
      }
      frame #15 {
        w213 = "Data: Initialize\nInitialize Core Data\nUI: Initialize\nUI: Front Panel State >> Open\nInit_Serial"  # Data: Initialize Initialize Core Data UI: Initialize UI: Front Panel State >> Open Init_Serial
        # "Initialization Macro\n(This is called once, when the VI starts)"
        n74 = call <vilib>:"Add State(s) to Queue__jki_lib_state_machine.vi"("State(s) in Front (\"\")"=w213, "State(s) in (\"\")"=w217) -> ("States Out"=w216:string)  [unwired: 13 in]
      }
      frame #16 {
        # "Exit Macro\n(This is called once, when the VI exits)"
        n75 = disable-structure shown="Enabled" {
          disable-tunnel: w219 -> [w229 _]
          disable-tunnel: [w223 _] -> w218
          frame #0 {
            n76 = Unbundle By Name(w229) -> ("Core.Close Panel on Exit?"=w228:bool)
            n77 = Select(t="UI: Front Panel State >> Close", s=w228, f="") -> (s? t:f=w225:string)
            n78 = call <vilib>:"Add State(s) to Queue__jki_lib_state_machine.vi"("State(s) in (\"\")"=w225, "State(s) at Back (\"\")"="Data: Cleanup\nExit") -> ("States Out"=w223:string)  [unwired: 13 in]
          }
          frame #1 {
          }
        }
        n79 = call <vilib>:"Add State(s) to Queue__jki_lib_state_machine.vi"("State(s) in Front (\"\")"=w218, "State(s) in (\"\")"=w222) -> ("States Out"=w221:string)  [unwired: 13 in]
      }
      frame #17 {
        # "Template Separator\n(You can make a copy of, or modify, this frame)"
        n80 = call <vilib>:"Add State(s) to Queue__jki_lib_state_machine.vi"("State(s) in (\"\")"=w233) -> ("States Out"=w232:string)  [unwired: 14 in]
      }
      frame #18 {
        # "Your code here.\n(You can make a copy of, or modify, this frame)"
        n81 = case shown="True" "InitSerial?" {
          tunnel: [w247 w269] -> w240
          tunnel: w239 -> [w246 w279]
          tunnel: [w245 w278] -> w238
          tunnel: w237 -> [w252 w272]
          tunnel: w236 -> [_ _]
          tunnel: [w244 w270] -> w234
          frame #0 {
            # "skip error handle routine"
            n82 = Unbundle By Name(w246) -> ("ComPort"=w243:refnum<visa-resource-name>)
            n83 = property class="Instr"(reference=w243) -> (reference out=w249:refnum<visa-resource-name>, "Serial Settings:Number of Bytes at Serial Port"=w251:u32)  [unwired: 1 in, 1 out]
            n84 = Greater Than 0?(x=w251) -> (x > 0?=w250:bool)
            n85 = case shown="True" w250 {
              tunnel: w252 -> [w265 w268]
              tunnel: [w265 w267] -> w248
              tunnel: w249 -> [_ w266]
              frame #0 {
              }
              frame #1 {
                n86 = VISA Clear(VISA resource name=w266, error in (no error)=w268) -> (error out=w267:errorcluster)  [unwired: 1 out]
              }
            }
            n87 = case shown="No Error" w248 {
              selector: w248 -> [w253 w260]
              tunnel: w246 -> [w257 w264]
              tunnel: [w256 w263] -> w245
              tunnel: w243 -> [w255 _]
              tunnel: ["" ("State(s) in Front (\"\")") "Macro: Exit" ("State(s) in Front (\"\")")] -> w244
              tunnel: [w253 w259] -> w247
              frame #0 {
                n88 = Bundle By Name(cluster=w257, "ComPort"=w255) -> (w256:T5)
              }
              frame #1 {
                n89 = Bundle By Name(cluster=w264, "Error Out Flag"=TRUE) -> (w263:T5)
                n90 = Bundle By Name(cluster=w260, "status"=FALSE) -> (w259:errorcluster)
              }
            }
          }
          frame #1 {
            # "skip error handle routine"
            # "Assumes that if the serial port is 19200, then it is all ok."
            n91 = Unbundle By Name(w279) -> ("ComPort"=w277:refnum<visa-resource-name>)
            n92 = disable-structure shown="Enabled" {
              disable-tunnel: w277 -> [w315 _]
              disable-tunnel: [w312 TRUE] -> w276
              frame #0 {
                n93 = property class="Instr"(reference=w315) -> ("Baud"=w314:u32)  [unwired: 1 in, 2 out]
                n94 = Not Equal?(x=w314, y=u32 19200) -> (x != y?=w312:bool)
              }
              frame #1 {
              }
            }
            n95 = case shown="True" w276 {
              tunnel: [w317 w320] -> w275
              tunnel: [w318 w319] -> w273
              tunnel: w272 -> [w317 w322]
              tunnel: w277 -> [w318 w321]
              frame #0 {
              }
              frame #1 {
                w328 = u16 0 items=["None", "XON/XOFF", "RTS/CTS", "XON/XOFF & RTS/CTS", "DTR/DSR", "XON/XOFF & DTR/DSR"] ("flow control (0:none)")
                w327 = u16 10 items=["1.0"=10, "1.5"=15, "2.0"=20] ("stop bits (10: 1 bit)")
                n96 = call-poly "VISA Configure Serial Port"("VISA resource name"=w321, "timeout (10sec)"=u32 1000, "Enable Termination\nChar (T)"=FALSE ("Enable Termination\nChar (T)"), "baud rate (9600)"=u32 19200, "data bits (8)"=u16 8, "parity (0:none)"=enum16{"None", "Odd", "Even", "Mark", "Space"}."None", "error in (no error)"=w322, "stop bits (10: 1 bit)"=w327, "flow control (0:none)"=w328) -> ("VISA resource name out"=w319:refnum<visa-resource-name>, "error out"=w320:errorcluster)  [unwired: 5 in]
              }
            }
            n97 = disable-structure shown="Enabled" {
              disable-tunnel: w275 -> [w297 w311]
              disable-tunnel: [w296 w310] -> w271
              disable-tunnel: [w295 w309] -> w274
              disable-tunnel: w273 -> [w294 w309]
              frame #0 {
                n98 = disable-structure shown="Enabled" {
                  disable-tunnel: w294 -> [w300 w302]
                  disable-tunnel: [w299 w302] -> w293
                  disable-tunnel: [w298 u32 1 ("Bytes at Port")] -> w292
                  frame #0 {
                    n99 = property class="Instr"(reference=w300) -> (reference out=w299:refnum<visa-resource-name>, "Serial Settings:Number of Bytes at Serial Port"=w298:u32)  [unwired: 1 in, 1 out]
                  }
                  frame #1 {
                  }
                }
                n100 = case shown="1, Default" w292 {
                  tunnel: w297 -> [w304 w308]
                  tunnel: [w304 w307] -> w296
                  tunnel: [w303 w306] -> w295
                  tunnel: w293 -> [w303 w305]
                  frame #0 {
                  }
                  frame #1 {
                    n101 = VISA Clear(VISA resource name=w305, error in (no error)=w308) -> (VISA resource name out=w306:refnum<visa-resource-name>, error out=w307:errorcluster)
                  }
                }
              }
              frame #1 {
                n102 = VISA Flush I/O Buffer(VISA resource name=w309, error in (no error)=w311) -> (error out=w310:errorcluster)  [unwired: 1 in, 1 out]
              }
            }
            n103 = case shown="Error" w271 {
              selector: w271 -> [w280 w287]
              tunnel: w279 -> [w284 w291]
              tunnel: [w283 w290] -> w278
              tunnel: w274 -> [w282 _]
              tunnel: ["" ("State(s) in Front (\"\")") "Macro: Exit" ("State(s) in Front (\"\")")] -> w270
              tunnel: [w280 w285] -> w269
              frame #0 {
                n104 = Bundle By Name(cluster=w284, "ComPort"=w282) -> (w283:T5)
              }
              frame #1 {
                n105 = Bundle By Name(cluster=w291, "Error Out Flag"=TRUE) -> (w290:T5)
                n106 = Bundle By Name(cluster=w287, "status"=FALSE) -> (w285:errorcluster)
              }
            }
          }
        }
        n107 = call <vilib>:"Add State(s) to Queue__jki_lib_state_machine.vi"("State(s) in Front (\"\")"=w234, "State(s) in (\"\")"=w242) -> ("States Out"=w241:string)  [unwired: 13 in]
      }
      frame #19 {
        w345 = u8 227  # ETX
        w348 = u8 226  # STX
        n108 = Unbundle By Name(w334) -> ("ComPort"=w358:refnum<visa-resource-name>)
        n109 = call "HEWH_DSM_CMD.vi"("Command"="Command") -> ("CMD Array"=w350:u8[])  [unwired: 10 in]
        n110 = Array Size(array=w350) -> (size(s)=w356:i32)
        n111 = Array Size(array="Command Data") -> (size(s)=w354:i32)
        n112 = Compound Arithmetic op=ADD(7 ("x"), w356, w354) -> (w352:i32)
        n113 = To Unsigned Byte Integer(number=w352) -> (unsigned 8bit integer=w353:u8)
        n114 = Build Array (concatenate)("Destination Address", w353, "Source Address", w350, "Command Data") -> (w347:u8[])
        n115 = call "crc16-ccitt (x1021).vi"("unsigned byte array"=w347) -> ("CRC"=w346:u8[])  [unwired: 9 in, 1 out]
        n116 = Build Array (concatenate)(w348, w347, w346, w345) -> (w339:u8[])
        "Command" <- w339
        n117 = flat-sequence {
          tunnel: [w380] -> w337
          tunnel: w336 -> [_]
          frame #0 {
            n118 = Tick Count (ms)() -> (millisecond timer value=w380:u32)
          }
        }
        n119 = Bundle By Name(cluster=w334, "HEWH Command"="Command") -> (w333:T5)
        n120 = disable-structure shown="Enabled" {
          disable-tunnel: w358 -> [w366 w372]
          disable-tunnel: w336 -> [w365 w371]
          disable-tunnel: [w364 w370] -> w344
          disable-tunnel: [w363 w369] -> w342
          disable-tunnel: w339 -> [w361 w368]
          disable-tunnel: w337 -> [_ w367]
          frame #0 {
            n121 = Byte Array To String(unsigned byte array=w361) -> (string=w362:string)
            n122 = VISA Write(VISA resource name=w366, write buffer=w362, error in (no error)=w365) -> (VISA resource name out=w364:refnum<visa-resource-name>, error out=w363:errorcluster)  [unwired: 1 out]
          }
          frame #1 {
            n123 = for {
              tunnel: w372 -> [w379]
              tunnel: w371 -> [w378]
              tunnel: w368 -> [w377] mode=indexing
              tunnel: [w376] -> w370
              tunnel: [w374] -> w369
              tunnel: w367 -> [_]
              n124 = Build Array(w377) -> (w373:u8[])
              n125 = Byte Array To String(unsigned byte array=w373) -> (string=w375:string)
              n126 = VISA Write(VISA resource name=w379, write buffer=w375, error in (no error)=w378) -> (VISA resource name out=w376:refnum<visa-resource-name>, error out=w374:errorcluster)  [unwired: 1 out]
            }
          }
        }
        n127 = Array Size(array=w339) -> (size(s)=w340:i32)
        n128 = Byte Array To String(unsigned byte array=w339) -> (string=w338:string)
        n129 = VISA Read(VISA resource name=w344, byte count=w340, error in (no error)=w342) -> (read buffer=w343:string, error out=w335:errorcluster)  [unwired: 2 out]
        n130 = Equal?(x=w338, y=w343) -> (x = y?=→"WriteOK":bool)
        n131 = call "Delay mS.vi"("Error In"=w335, "milliseconds to wait"=u32 10) -> ("Error Out"=w331:errorcluster)  [unwired: 13 in]
        n132 = call <vilib>:"Add State(s) to Queue__jki_lib_state_machine.vi"("State(s) in (\"\")"=w360) -> ("States Out"=w359:string)  [unwired: 14 in]
        "tStart" <- w337
      }
      frame #20 {
        # "Your code here.\n(You can make a copy of, or modify, this frame)"
        n133 = Unbundle By Name(w387) -> ("ComPort"=w386:refnum<visa-resource-name>)
        n134 = for {
          tunnel: w386 -> [w400]
          tunnel: "Random Data" -> [w396] mode=indexing
          tunnel: [w393] -> w385 mode=indexing
          shift-right: [w392] -> w383
          shift-left: w384 -> [w391]
          n135 = Build Array(w396) -> (w397:u8[])
          n136 = Byte Array To String(unsigned byte array=w397) -> (string=w394:string)
          n137 = VISA Write(VISA resource name=w400, write buffer=w394, error in (no error)=w391) -> (VISA resource name out=w399:refnum<visa-resource-name>, error out=w390:errorcluster)  [unwired: 1 out]
          n138 = VISA Read(VISA resource name=w399, byte count=u32 1, error in (no error)=w390) -> (read buffer=w395:string, error out=w392:errorcluster)  [unwired: 2 out]
          n139 = Equal?(x=w394, y=w395) -> (x = y?=w393:bool)
        }
        n140 = And Array Elements(Boolean array=w385) -> (logical AND=w381:bool)
        n141 = local write "WriteOK"(w381) -> ()
        n142 = call <vilib>:"Add State(s) to Queue__jki_lib_state_machine.vi"("State(s) in (\"\")"=w389) -> ("States Out"=w388:string)  [unwired: 14 in]
      }
      frame #21 {
        # "Template Separator\n(You can make a copy of, or modify, this frame)"
        n143 = call <vilib>:"Add State(s) to Queue__jki_lib_state_machine.vi"("State(s) in (\"\")"=w404) -> ("States Out"=w403:string)  [unwired: 14 in]
      }
      frame #22 {
        # "Your code here.\n(You can make a copy of, or modify, this frame)"
        n144 = case shown="False" FALSE {
          tunnel: w407 -> [_ w420]
          tunnel: [u8[] [] ("unsigned byte array") w418] -> w406
          frame #0 {
          }
          frame #1 {
            n145 = Unbundle By Name(w420) -> ("ComPort"=w417:refnum<visa-resource-name>)
            n146 = while {
              tunnel: w417 -> [w429]
              shift-right: [w421] -> _
              shift-left: u32 1000000 ("Serial Settings:Number of Bytes at Serial Port 5") -> [w428]
              tunnel: [w421] -> w415
              i -> [w426]
              stop <- w424 stop-if-true
              n147 = property class="Instr"(reference=w429) -> ("Serial Settings:Number of Bytes at Serial Port"=w421:u32)  [unwired: 1 in, 2 out]
              n148 = Not Equal?(x=0, y=w426) -> (x != y?=w422:bool)
              n149 = Equal?(x=w428, y=w421) -> (x = y?=w423:bool)
              n150 = And(x=w423, y=w422) -> (x .and. y?=w424:bool)
              n151 = Wait (ms)(milliseconds to wait="milliseconds to wait") -> ()  [unwired: 1 out]
              "Numeric" <- w426
            }
            "byte count" <- w415
            n152 = VISA Read(VISA resource name=w417, byte count=w415) -> (read buffer=w419:string)  [unwired: 1 in, 3 out]
            n153 = String To Byte Array(string=w419) -> (unsigned byte array=w418:u8[])
            n154 = local write "ReadArray"(w418) -> ()
          }
        }
        n155 = Bundle By Name(cluster=w407, "ReadArray"=w406, "CRCArray"=u8[] [] ("ReadArray")) -> (w410:T5)
        n156 = call <vilib>:"Add State(s) to Queue__jki_lib_state_machine.vi"("State(s) in Front (\"\")"="ReadData: ACK" ("State(s) in Front (\"\")"), "State(s) in (\"\")"=w413) -> ("States Out"=w412:string)  [unwired: 13 in]
      }
      frame #23 {
        w434 = u8 225  # ACK
        # "Read ACK Byte"
        n157 = Unbundle By Name(w446) -> ("ComPort"=w432:refnum<visa-resource-name>, "ReadArray"=w433:u8[], "HEWH Command"=w430:u8)  [unwired: 1 out]
        n158 = local write "ReadArray"(w433) -> ()
        n159 = VISA Read(VISA resource name=w432, byte count=u32 1, error in (no error)=w439) -> (read buffer=w443:string, error out=w437:errorcluster)  [unwired: 2 out]
        n160 = property class="Instr"(reference=w432) -> ("Serial Settings:Number of Bytes at Serial Port"=→"Serial Settings:Number of Bytes at Serial Port 2":u32)  [unwired: 1 in, 2 out]
        n161 = String To Byte Array(string=w443) -> (unsigned byte array=w442:u8[])
        n162 = Index Array(array=w442, index=0) -> (element=w440:u8)
        n163 = Build Array (concatenate)(w433, w442) -> (w447:u8[])
        n164 = Equal?(x=w440, y=w434) -> (x = y?=w438:bool)
        "WriteACK" <- w438
        n165 = Bundle By Name(cluster=w446, "ReadArray"=w447) -> (w445:T5)
        n166 = case shown="True" w438 {
          tunnel: w437 -> [w452 w457]
          tunnel: [w450 w457] -> w436
          tunnel: ["ReadData: Rest" ("State(s) in Front (\"\")") w456] -> w435
          tunnel: w430 -> [_ w455]
          frame #0 {
            n167 = call "Error Bool Enumerator.vi"("Error Enum"=HEWH_Error_Enumeration."GEA2 ReadACK", "Error In"=w452) -> ("Error Out"=w450:errorcluster)  [unwired: 7 in]
          }
          frame #1 {
            n168 = call "HEWH Command Needs Read.vi"("Command"=w455) -> ("RQST"=w454:bool)  [unwired: 13 in, 1 out]
            n169 = case shown="True" w454 {
              tunnel: ["ReadData: STX" ("State(s) in Front (\"\")") "Macro: Exit" ("State(s) in Front (\"\")")] -> w456
              frame #0 {
              }
              frame #1 {
              }
            }
          }
        }
        n170 = call <vilib>:"Add State(s) to Queue__jki_lib_state_machine.vi"("State(s) in Front (\"\")"=w435, "State(s) in (\"\")"=w449) -> ("States Out"=w448:string)  [unwired: 13 in]
      }
      frame #24 {
        w469 = u8 224  # ESC
        # "Read Destination byte.  If its your message, than continue to length, otherwise, read the rest of the message."
        n171 = Unbundle By Name(w482) -> ("ComPort"=w462:refnum<visa-resource-name>, "ReadArray"=w460:u8[])
        n172 = VISA Read(VISA resource name=w462, byte count=u32 1, error in (no error)=w476) -> (read buffer=w479:string, error out=w464:errorcluster)  [unwired: 2 out]
        n173 = String To Byte Array(string=w479) -> (unsigned byte array=w466:u8[])
        n174 = Index Array(array=w466, index=0) -> (element=w471:u8)
        n175 = local write "ReadArray"(w460) -> ()
        n176 = Equal?(x=w471, y=w469) -> (x = y?=w468:bool)
        n177 = case shown="True" w468 {
          tunnel: [w487 w488] -> w467
          tunnel: w466 -> [w487 w495]
          tunnel: [w486 w489] -> w465
          tunnel: w460 -> [w486 w496]
          tunnel: w464 -> [w485 w492]
          tunnel: [w485 w491] -> w463
          tunnel: w462 -> [_ w490]
          frame #0 {
          }
          frame #1 {
            n178 = VISA Read(VISA resource name=w490, byte count=u32 1, error in (no error)=w492) -> (read buffer=w494:string, error out=w491:errorcluster)  [unwired: 2 out]
            n179 = String To Byte Array(string=w494) -> (unsigned byte array=w488:u8[])
            n180 = Build Array (concatenate)(w496, w495) -> (w489:u8[])
          }
        }
        n181 = Build Array (concatenate)(w465, w467) -> (w461:u8[])
        n182 = local read "Source Address"() -> (w472:u8)
        n183 = Index Array(array=w467, index=0) -> (element=w477:u8)
        n184 = Bundle By Name(cluster=w482, "ReadArray"=w461, "CRCArray"=w467) -> (w481:T5)
        n185 = Equal?(x=w477, y=w472) -> (x = y?=w475:bool)
        n186 = case shown="False" w475 {
          tunnel: w463 -> [w500 w502]
          tunnel: [w498 w502] -> w474
          tunnel: ["ReadData: Rest" ("State(s) in Front (\"\")") "ReadData: Length" ("State(s) in Front (\"\")")] -> w473
          frame #0 {
            n187 = call <vilib>:"Merge Errors.vi"("error in 2 (no error)"=errorcluster {"status"=FALSE, "code"=7000, "source"="Message not for Me"}, "error in 1 (no error)"=w500) -> ("error out"=w498:errorcluster)  [unwired: 5 in]
          }
          frame #1 {
          }
        }
        n188 = call <vilib>:"Add State(s) to Queue__jki_lib_state_machine.vi"("State(s) in Front (\"\")"=w473, "State(s) in (\"\")"=w484) -> ("States Out"=w483:string)  [unwired: 13 in]
      }
      frame #25 {
        w517 = u8 224  # ESC
        # "Your code here.\n(You can make a copy of, or modify, this frame)"
        n189 = Unbundle By Name(w528) -> ("ComPort"=w511:refnum<visa-resource-name>, "ReadArray"=w509:u8[], "CRCArray"=w503:u8[])
        n190 = VISA Read(VISA resource name=w511, byte count=u32 1, error in (no error)=w523) -> (read buffer=w525:string, error out=w513:errorcluster)  [unwired: 2 out]
        n191 = String To Byte Array(string=w525) -> (unsigned byte array=w515:u8[])
        n192 = local write "ReadArray"(w509) -> ()
        n193 = Index Array(array=w515, index=0) -> (element=w519:u8)
        n194 = Equal?(x=w519, y=w517) -> (x = y?=w516:bool)
        n195 = case shown="True" w516 {
          tunnel: [w534 w535] -> w504
          tunnel: w515 -> [w534 w542]
          tunnel: [w533 w536] -> w514
          tunnel: w509 -> [w533 w543]
          tunnel: w513 -> [w532 w539]
          tunnel: [w532 w538] -> w512
          tunnel: w511 -> [_ w537]
          frame #0 {
          }
          frame #1 {
            n196 = VISA Read(VISA resource name=w537, byte count=u32 1, error in (no error)=w539) -> (read buffer=w541:string, error out=w538:errorcluster)  [unwired: 2 out]
            n197 = String To Byte Array(string=w541) -> (unsigned byte array=w535:u8[])
            n198 = Build Array (concatenate)(w543, w542) -> (w536:u8[])
          }
        }
        n199 = Index Array(array=w504, index=0) -> (element=w508:u8)
        n200 = Build Array (concatenate)(w514, w504) -> (w529:u8[])
        n201 = Subtract(x=w508, y=u8 6) -> (x-y=w506:u8)
        n202 = Build Array (concatenate)(w503, w504) -> (w505:u8[])
        n203 = Less Or Equal?(x=w506, y=u8 0 ("0")) -> (x <= y?=w522:bool)
        n204 = Bundle By Name(cluster=w528, "ReadArray"=w529, "CRCArray"=w505, "Bytes Remaining"=w506) -> (w527:T5)
        n205 = case shown="False" w522 {
          tunnel: w512 -> [w545 w549]
          tunnel: [w545 w547] -> w521
          tunnel: ["ReadData: Bytes" ("State(s) in Front (\"\")") "ReadData: Rest" ("State(s) in Front (\"\")")] -> w520
          frame #0 {
          }
          frame #1 {
            n206 = call <vilib>:"Merge Errors.vi"("error in 2 (no error)"=errorcluster {"status"=FALSE, "code"=7000, "source"="0 Length"}, "error in 1 (no error)"=w549) -> ("error out"=w547:errorcluster)  [unwired: 5 in]
          }
        }
        n207 = call <vilib>:"Add State(s) to Queue__jki_lib_state_machine.vi"("State(s) in Front (\"\")"=w520, "State(s) in (\"\")"=w531) -> ("States Out"=w530:string)  [unwired: 13 in]
      }
      frame #26 {
        w563 = u8 224  # ESC
        # "Your code here.\n(You can make a copy of, or modify, this frame)"
        n208 = Unbundle By Name(w572) -> ("ComPort"=w557:refnum<visa-resource-name>, "ReadArray"=w553:u8[], "Bytes Remaining"=w555:u8, "CRCArray"=w550:u8[])
        n209 = VISA Read(VISA resource name=w557, byte count=u32 1, error in (no error)=w568) -> (read buffer=w569:string, error out=w559:errorcluster)  [unwired: 2 out]
        n210 = String To Byte Array(string=w569) -> (unsigned byte array=w561:u8[])
        n211 = Index Array(array=w561, index=0) -> (element=w565:u8)
        n212 = Equal?(x=w565, y=w563) -> (x = y?=w562:bool)
        n213 = case shown="True" w562 {
          tunnel: [w578 w579] -> w552
          tunnel: w561 -> [w578 w586]
          tunnel: [w577 w580] -> w560
          tunnel: w553 -> [w577 w587]
          tunnel: w559 -> [w576 w583]
          tunnel: [w576 w582] -> w558
          tunnel: w557 -> [_ w581]
          frame #0 {
          }
          frame #1 {
            n214 = VISA Read(VISA resource name=w581, byte count=u32 1, error in (no error)=w583) -> (read buffer=w585:string, error out=w582:errorcluster)  [unwired: 2 out]
            n215 = String To Byte Array(string=w585) -> (unsigned byte array=w579:u8[])
            n216 = Build Array (concatenate)(w587, w586) -> (w580:u8[])
          }
        }
        n217 = local write "ReadArray"(w553) -> ()
        n218 = Decrement(x=w555) -> (x-1=w554:u8)
        n219 = Build Array (concatenate)(w550, w552) -> (w551:u8[])
        n220 = Build Array (concatenate)(w560, w552) -> (w573:u8[])
        n221 = Greater Than 0?(x=w554) -> (x > 0?=w556:bool)
        n222 = Bundle By Name(cluster=w572, "ReadArray"=w573, "CRCArray"=w551, "Bytes Remaining"=w554) -> (w571:T5)
        n223 = case shown="True" w556 {
          tunnel: w558 -> [w591 w593]
          tunnel: [w589 w593] -> w567
          tunnel: ["ReadData: CRC1" ("State(s) in Front (\"\")") "ReadData: Bytes" ("State(s) in Front (\"\")")] -> w566
          frame #0 {
            n224 = call <vilib>:"Merge Errors.vi"("error in 2 (no error)"=errorcluster {"status"=FALSE, "code"=7000, "source"="0 Length"}, "error in 1 (no error)"=w591) -> ("error out"=w589:errorcluster)  [unwired: 5 in]
          }
          frame #1 {
          }
        }
        n225 = call <vilib>:"Add State(s) to Queue__jki_lib_state_machine.vi"("State(s) in Front (\"\")"=w566, "State(s) in (\"\")"=w575) -> ("States Out"=w574:string)  [unwired: 13 in]
      }
      frame #27 {
        w602 = u8 224  # ESC
        # "Your code here.\n(You can make a copy of, or modify, this frame)"
        n226 = Unbundle By Name(w610) -> ("ComPort"=w596:refnum<visa-resource-name>, "ReadArray"=w598:u8[])
        n227 = VISA Read(VISA resource name=w596, byte count=u32 1, error in (no error)=w606) -> (read buffer=w607:string, error out=w597:errorcluster)  [unwired: 2 out]
        n228 = String To Byte Array(string=w607) -> (unsigned byte array=w600:u8[])
        n229 = Index Array(array=w600, index=0) -> (element=w604:u8)
        n230 = Equal?(x=w604, y=w602) -> (x = y?=w601:bool)
        n231 = case shown="True" w601 {
          tunnel: [w616 w617] -> w595
          tunnel: w600 -> [w616 w624]
          tunnel: [w615 w618] -> w599
          tunnel: w598 -> [w615 w625]
          tunnel: w597 -> [w614 w621]
          tunnel: [w614 w620] -> w594
          tunnel: w596 -> [_ w619]
          frame #0 {
          }
          frame #1 {
            n232 = VISA Read(VISA resource name=w619, byte count=u32 1, error in (no error)=w621) -> (read buffer=w623:string, error out=w620:errorcluster)  [unwired: 2 out]
            n233 = String To Byte Array(string=w623) -> (unsigned byte array=w617:u8[])
            n234 = Build Array (concatenate)(w625, w624) -> (w618:u8[])
          }
        }
        n235 = Build Array (concatenate)(w599, w595) -> (w611:u8[])
        n236 = Bundle By Name(cluster=w610, "ReadArray"=w611, "CRCRead"=w595) -> (w609:T5)
        n237 = call <vilib>:"Add State(s) to Queue__jki_lib_state_machine.vi"("State(s) in Front (\"\")"="ReadData: CRC2" ("State(s) in Front (\"\")"), "State(s) in (\"\")"=w613) -> ("States Out"=w612:string)  [unwired: 13 in]
      }
      frame #28 {
        w637 = u8 224  # ESC
        # "Your code here.\n(You can make a copy of, or modify, this frame)"
        n238 = Unbundle By Name(w645) -> ("ComPort"=w632:refnum<visa-resource-name>, "ReadArray"=w628:u8[], "CRCRead"=w627:u8[])
        n239 = VISA Read(VISA resource name=w632, byte count=u32 1, error in (no error)=w641) -> (read buffer=w642:string, error out=w633:errorcluster)  [unwired: 2 out]
        n240 = String To Byte Array(string=w642) -> (unsigned byte array=w635:u8[])
        n241 = Index Array(array=w635, index=0) -> (element=w639:u8)
        n242 = Equal?(x=w639, y=w637) -> (x = y?=w636:bool)
        n243 = case shown="True" w636 {
          tunnel: [w650 w651] -> w629
          tunnel: w635 -> [w650 w658]
          tunnel: [w649 w652] -> w634
          tunnel: w628 -> [w649 w659]
          tunnel: w633 -> [w648 w655]
          tunnel: [w648 w654] -> w631
          tunnel: w632 -> [_ w653]
          frame #0 {
          }
          frame #1 {
            n244 = VISA Read(VISA resource name=w653, byte count=u32 1, error in (no error)=w655) -> (read buffer=w657:string, error out=w654:errorcluster)  [unwired: 2 out]
            n245 = String To Byte Array(string=w657) -> (unsigned byte array=w651:u8[])
            n246 = Build Array (concatenate)(w659, w658) -> (w652:u8[])
          }
        }
        n247 = local write "ReadArray"(w628) -> ()
        n248 = Build Array (concatenate)(w634, w629) -> (w630:u8[])
        n249 = Build Array (concatenate)(w627, w629) -> (w626:u8[])
        n250 = Bundle By Name(cluster=w645, "ReadArray"=w630, "CRCRead"=w626) -> (w644:T5)
        n251 = local write "CRCRead"(w626) -> ()
        n252 = call <vilib>:"Add State(s) to Queue__jki_lib_state_machine.vi"("State(s) in Front (\"\")"="ReadData: CheckCRC" ("State(s) in Front (\"\")"), "State(s) in (\"\")"=w647) -> ("States Out"=w646:string)  [unwired: 13 in]
      }
      frame #29 {
        # "Your code here.\n(You can make a copy of, or modify, this frame)"
        n253 = Unbundle By Name(w662) -> ("CRCRead"=w667:u8[], "CRCArray"=w664:u8[])
        "DataReturned" <- w664
        n254 = call "crc16-ccitt (x1021).vi"("error in (no error)"=w668, "unsigned byte array"=w664) -> ("error out (dup)"=w665:errorcluster, "CRC"=w663:u8[])  [unwired: 8 in]
        n255 = Equal?(x=w667, y=w663) -> (x = y?=w660:bool)
        "CRC Match" <- w660
        n256 = case shown="True" w660 {
          tunnel: ["ReadData: Rest" ("State(s) in Front (\"\")") "ReadData: ETX" ("State(s) in Front (\"\")")] -> w669
          tunnel: [w675 w677] -> w666
          tunnel: w665 -> [w674 w677]
          frame #0 {
            n257 = call "Error Bool Enumerator.vi"("Error Enum"=HEWH_Error_Enumeration."GEA2 CRC Mismatch", "Error In"=w674, "Error?"=TRUE) -> ("Error Out"=w675:errorcluster)  [unwired: 6 in]
          }
          frame #1 {
          }
        }
        n258 = Bundle By Name(cluster=w662, "CRC"=w660) -> (w661:T5)
        n259 = call <vilib>:"Add State(s) to Queue__jki_lib_state_machine.vi"("State(s) in Front (\"\")"=w669, "State(s) in (\"\")"=w671) -> ("States Out"=w670:string)  [unwired: 13 in]
      }
      frame #30 {
        w685 = u8 226  # STX
        # "Your code here.\n(You can make a copy of, or modify, this frame)"
        n260 = Unbundle By Name(w681) -> ("ComPort"=w680:refnum<visa-resource-name>, "ReadArray"=w698:u8[])
        n261 = property class="Instr"(reference=w680) -> (reference out=w679:refnum<visa-resource-name>, "Serial Settings:Number of Bytes at Serial Port"=→"Serial Settings:Number of Bytes at Serial Port 4":u32)  [unwired: 1 in, 1 out]
        n262 = VISA Read(VISA resource name=w679, byte count=u32 1, error in (no error)=w695) -> (VISA resource name out=w683:refnum<visa-resource-name>, read buffer=w689:string, error out=w693:errorcluster)  [unwired: 1 out]
        n263 = String To Byte Array(string=w689) -> (unsigned byte array=w688:u8[])
        n264 = property class="Instr"(reference=w683) -> ("Serial Settings:Number of Bytes at Serial Port"=→"Serial Settings:Number of Bytes at Serial Port 3":u32)  [unwired: 1 in, 2 out]
        n265 = Index Array(array=w688, index=0) -> (element=w686:u8)
        n266 = Build Array (concatenate)(w698, w688) -> (w697:u8[])
        n267 = Equal?(x=w686, y=w685) -> (x = y?=w694:bool)
        n268 = case shown="False" w694 {
          tunnel: w693 -> [w704 w707]
          tunnel: [w701 w707] -> w692
          tunnel: ["ReadData: Rest" ("State(s) in Front (\"\")") "ReadData: Destination" ("State(s) in Front (\"\")")] -> w691
          frame #0 {
            n269 = call "Error Bool Enumerator.vi"("Error Enum"=HEWH_Error_Enumeration."GEA2 STX", "Error In"=w704, "Error?"=TRUE) -> ("Error Out"=w701:errorcluster)  [unwired: 6 in]
          }
          frame #1 {
          }
        }
        n270 = Bundle By Name(cluster=w681, "ReadArray"=w697) -> (w696:T5)
        n271 = call <vilib>:"Add State(s) to Queue__jki_lib_state_machine.vi"("State(s) in Front (\"\")"=w691, "State(s) in (\"\")"=w700) -> ("States Out"=w699:string)  [unwired: 13 in]
      }
      frame #31 {
        w708 = u8 227  # ETX
        # "Your code here.\n(You can make a copy of, or modify, this frame)"
        n272 = Unbundle By Name(w720) -> ("ComPort"=w723:refnum<visa-resource-name>, "ReadArray"=w722:u8[])
        n273 = VISA Read(VISA resource name=w723, byte count=u32 1, error in (no error)=w718) -> (read buffer=w712:string, error out=w716:errorcluster)  [unwired: 2 out]
        n274 = String To Byte Array(string=w712) -> (unsigned byte array=w711:u8[])
        n275 = Index Array(array=w711, index=0) -> (element=w709:u8)
        n276 = Build Array (concatenate)(w722, w711) -> (w721:u8[])
        n277 = Equal?(x=w709, y=w708) -> (x = y?=w717:bool)
        n278 = Bundle By Name(cluster=w720, "ReadArray"=w721) -> (w719:T5)
        n279 = case shown="False" w717 {
          tunnel: w716 -> [w728 w732]
          tunnel: [w730 w732] -> w715
          tunnel: ["ReadData: Rest" ("State(s) in Front (\"\")") "ReadData: SendACK" ("State(s) in Front (\"\")")] -> w714
          frame #0 {
            n280 = call "Error Bool Enumerator.vi"("Error Enum"=HEWH_Error_Enumeration."GEA2 ETX", "Error In"=w728, "Error?"=TRUE) -> ("Error Out"=w730:errorcluster)  [unwired: 6 in]
          }
          frame #1 {
          }
        }
        n281 = call <vilib>:"Add State(s) to Queue__jki_lib_state_machine.vi"("State(s) in Front (\"\")"=w714, "State(s) in (\"\")"=w725) -> ("States Out"=w724:string)  [unwired: 13 in]
      }
      frame #32 {
        n282 = Unbundle By Name(w743) -> ("ComPort"=w740:refnum<visa-resource-name>, "ReadArray"=w744:u8[])
        n283 = disable-structure shown="Enabled" {
          disable-tunnel: w740 -> [w749 w751]
          disable-tunnel: [w748 w751] -> w739
          disable-tunnel: [w747 u32 100 ("Bytes at Port")] -> w736
          frame #0 {
            n284 = property class="Instr"(reference=w749) -> (reference out=w748:refnum<visa-resource-name>, "Serial Settings:Number of Bytes at Serial Port"=w747:u32)  [unwired: 1 in, 1 out]
          }
          frame #1 {
          }
        }
        n285 = VISA Read(VISA resource name=w739, byte count=w736) -> (read buffer=w738:string, error out=w734:errorcluster)  [unwired: 1 in, 2 out]
        n286 = String To Byte Array(string=w738) -> (unsigned byte array=w737:u8[])
        n287 = Build Array (concatenate)(w744, w737) -> (w741:u8[])
        n288 = local write "ReadArray"(w741) -> ()
        n289 = Bundle By Name(cluster=w743, "ReadArray"=w741) -> (w742:T5)
        n290 = call <vilib>:"Merge Errors.vi"("error in 2 (no error)"=w734, "error in 1 (no error)"=w735) -> ("error out"=w733:errorcluster)  [unwired: 5 in]
        n291 = call <vilib>:"Add State(s) to Queue__jki_lib_state_machine.vi"("State(s) in (\"\")"=w746) -> ("States Out"=w745:string)  [unwired: 14 in]
      }
      frame #33 {
        w766 = u8 225  # ACK
        n292 = Unbundle By Name(w754) -> ("ReadArray"=w756:u8[], "ComPort"=w759:refnum<visa-resource-name>)
        n293 = property class="Instr"(reference=w759) -> ("Serial Settings:Number of Bytes at Serial Port"=→"Serial Settings:Number of Bytes at Serial Port":u32)  [unwired: 1 in, 2 out]
        n294 = Build Array(w766) -> (w769:u8[])
        n295 = Byte Array To String(unsigned byte array=w769) -> (string=w768:string)
        n296 = VISA Write(VISA resource name=w759, write buffer=w768, error in (no error)=w772) -> (VISA resource name out=w771:refnum<visa-resource-name>, error out=w767:errorcluster)  [unwired: 1 out]
        n297 = VISA Read(VISA resource name=w771, byte count=u32 1, error in (no error)=w767) -> (read buffer=w764:string, error out=w765:errorcluster)  [unwired: 2 out]
        n298 = Equal?(x=w768, y=w764) -> (x = y?=w762:bool)
        "Read_ACK" <- w762
        n299 = String To Byte Array(string=w764) -> (unsigned byte array=w755:u8[])
        "ACK(E1?)" <- w755
        n300 = Build Array (concatenate)(w756, w755) -> (w752:u8[])
        n301 = Not(x=w762) -> (.not. x?=w761:bool)
        n302 = local write "ReadArray"(w752) -> ()
        n303 = call "Error Bool Enumerator.vi"("Error Enum"=HEWH_Error_Enumeration."GEA2 Send ACK Mismatch", "Error In"=w765, "Error?"=w761) -> ("Error Out"=w757:errorcluster)  [unwired: 6 in]
        n304 = Bundle By Name(cluster=w754, "ReadArray"=w752) -> (w753:T5)
        n305 = case shown="No Error" w757 {
          tunnel: ["Macro: Exit" ("State(s) in Front (\"\")") "ReadData: Rest" ("State(s) in Front (\"\")")] -> w760
          frame #0 {
          }
          frame #1 {
          }
        }
        n306 = call <vilib>:"Add State(s) to Queue__jki_lib_state_machine.vi"("State(s) in Front (\"\")"=w760, "State(s) in (\"\")"=w774) -> ("States Out"=w773:string)  [unwired: 13 in]
      }
    }
    n307 = local write "Error Out"(w35) -> ()
    n308 = flat-sequence {
      tunnel: [w47] -> w34
      tunnel: w35 -> [_]
      tunnel: [w46] -> w33
      frame #0 {
        n309 = local read "tStart"() -> (w46:u32)
        n310 = Tick Count (ms)() -> (millisecond timer value=w47:u32)
      }
    }
    n311 = Build Array (concatenate)(w30, w29) -> (w28:string[])
    "State Array" <- w28
    n312 = To Long Integer(number=w34) -> (32bit integer=w32:i32)
    n313 = To Long Integer(number=w33) -> (32bit integer=w31:i32)
  }
  n314 = Subtract(x=w10, y=w9) -> (x-y=w11:i32[])
  "Time Array" <- w11
  n315 = Unbundle By Name(w2) -> ("ReadArray"=w7:u8[], "CRC"=w3:bool)
  n316 = Delete From Array(array=w11, length=1, index=0) -> (array with subset deleted=w13:i32[])  [unwired: 1 out]
  n317 = Unbundle By Name(w2) -> ("Error Out Flag"=w1:bool)
  n318 = for {
    tunnel: w13 -> [w779] mode=indexing
    tunnel: w11 -> [w778] mode=indexing
    tunnel: [w777] -> w12 mode=indexing
    n319 = Subtract(x=w779, y=w778) -> (x-y=w777:i32)
  }
  "Tdiff" <- w12
  n320 = local write "ReadArray"(w7) -> ()
  n321 = Bundle By Name(cluster=w16, "status"=w1) -> (w4:errorcluster)
  n322 = disable-structure shown="Enabled" {
    disable-tunnel: [w794 w798] -> w5
    disable-tunnel: w4 -> [w793 w798]
    disable-tunnel: w3 -> [w792 _]
    frame #0 {
      # "Patch for double read of ICP"
      n323 = call "Error Bool Enumerator.vi"("Error Enum"=HEWH_Error_Enumeration."GEA2 Send ACK Mismatch", "Error?"=TRUE) -> ("Error Out"=w781:errorcluster)  [unwired: 7 in]
      n324 = call "Error Bool Enumerator.vi"("Error Enum"=HEWH_Error_Enumeration."GEA2 ETX", "Error?"=TRUE) -> ("Error Out"=w783:errorcluster)  [unwired: 7 in]
      n325 = Unbundle By Name(w781) -> ("code"=w780:i32)
      n326 = Unbundle By Name(w783) -> ("code"=w782:i32)
      n327 = Unbundle By Name(w793) -> ("code"=w789:i32)
      n328 = Equal?(x=w789, y=w782) -> (x = y?=w790:bool)
      n329 = Equal?(x=w789, y=w780) -> (x = y?=w788:bool)
      n330 = Or(x=w790, y=w788) -> (x .or. y?=w791:bool)
      n331 = And(x=w792, y=w791) -> (x .and. y?=w795:bool)
      n332 = case shown="True" w795 {
        tunnel: [w796 errorcluster {"status"=FALSE, "code"=0, "source"="ETX or ACK"} ("Error Out")] -> w794
        tunnel: w793 -> [w796 _]
        frame #0 {
        }
        frame #1 {
        }
      }
    }
    frame #1 {
    }
  }
  "Error Out" <- w5
